vi "TDS - Thermal Desorption Spectroscopy.vi"() -> ()   [LabVIEW 2020]
uses:
  Control 2.ctl
  rga_lv_85/SRSRGA85.llb/SRSRGAo Units Enumeration.ctl
  TDS_ProccesConfig.ctl
  rga_lv_85/SRSRGA85.llb/SRSRGAo RefNum.ctl
  <vilib>/Utility/miscctls.llb/LVRowAndColumnTypeDef.ctl
  <vilib>/Utility/sysdir.llb/System Directory Type.ctl
  <vilib>/Modbus/master/Create Master Instance (TCP).vi
  <vilib>/Utility/config.llb/Read Key (String).vi
  <vilib>/Waveform/WDTFileIO.llb/Export Waveforms To Spreadsheet File (1D).vi
  <vilib>/Utility/config.llb/Write Key (String).vi
  <vilib>/Modbus/master/Modbus Master.lvclass
  <vilib>/Utility/config.llb/NI_LVConfig.lvlib
panel:
  in  "TDS 2":T1={"Target Temp:"=10.0, "Target Ramp:"=1.0, "Ramp unit:"=1, "Temp. unit:"=0, "Target Ue [V]:"=500.0, "Target Ic [A]:"=2.0, "Heating Mode:"=FALSE, "PID Output:"=FALSE, "Regulation Type"=FALSE, "RGA Specifications"=[{"Mass"=2, "Noise Floor"=4, "CEM "=FALSE}], "Heating Recipe"=[]} {"RGA Specifications"."Noise Floor" min=0 max=7; "RGA Specifications"."Mass" min=1 max=300; "Temp. unit:" items=["K"=1, "C"=0]; "Ramp unit:" items=["/s", "/m", "/h"]}
  in  "TDS":T1={"Target Temp:"=10.0, "Target Ramp:"=1.0, "Ramp unit:"=1, "Temp. unit:"=0, "Target Ue [V]:"=500.0, "Target Ic [A]:"=2.0, "Heating Mode:"=FALSE, "PID Output:"=FALSE, "Regulation Type"=FALSE, "RGA Specifications"=[{"Mass"=2, "Noise Floor"=4, "CEM "=FALSE}], "Heating Recipe"=[]} {"RGA Specifications"."Noise Floor" min=0 max=7; "RGA Specifications"."Mass" min=1 max=300; "Temp. unit:" items=["K"=1, "C"=0]; "Ramp unit:" items=["/s", "/m", "/h"]}
  in  "Reconnect":bool
  out "Remote:":bool
  out "RGA_LastData":sgl[](array[numeric]) format="%.2f"
  out "heat_LastData":dbl[](array[numeric])
  out "size(s) 3":i32
  out "HEAT start time":timestamp=timestamp(3621395400.2120705 s since 1904-01-01)
  out "Label.Text":string="D"
  out "Array 2":waveform(dbl)[](array[waveform])
  out "output array":sgl[][](array[numeric])=[[8.752041e-08, 0.0, 0.0, 0.0]]
  out "size(s)":i32=5
  out "Boolean":T2=TRUE
  out "output cluster":T3={"Time"=[0.0, 2.0, 4.0, 6.0, 8.0, 10.0, 12.0, 14.0, 16.0], "Temp"=[24.090000000000032, 10.0, 10.0, 20.0, 20.0, 30.0, 30.0, 40.0, 40.0], "Ramp"=[60.0, 7.045000000000016, 60.0, 5.0, 60.0, 5.0, 60.0, 5.0, 60.0]}
  out "StartTime":timestamp=timestamp(3621394478.675983 s since 1904-01-01)
  out "stopped_loops":bool=TRUE
  in  "Tab Control":T4(tab)
  in  "Start 1":bool=TRUE
  in  "Clear ALL":bool
  out "Waveform Graph":waveform(dbl)[](graph)=[{"t0"=timestamp(3717656497.7127247 s since 1904-01-01), "dt"=0.2, "Y"=array[417 elements]}, {"t0"=timestamp(3717656497.7127247 s since 1904-01-01), "dt"=0.2, "Y"=array[417 elements]}, {"t0"=timestamp(3717656497.7127247 s since 1904-01-01), "dt"=0.2, "Y"=[0.0, 0.0, 0.0, 0.0, 0.0, 0.0, 0.0, 0.0, 0.0, 0.0, 0.0, 0.0, 0.0, 0.0, 0.0, 0.0, 0.0, 0.0, 0.0, 0.0, 0.0, 0.0, 0.0, 0.0, 0.0, 0.0, 0.0, 0.0, 0.0, 0.0, 0.0, 0.0, 0.0, 0.0, 0.0, 0.0, 0.0, 0.0, 0.0, 0.0, 0.0, 0.0, 0.0, 0.0, 0.0, 0.0, 0.0, 0.0, 0.0, 0.0, 0.0, 0.0, 0.0, 0.0, 0.0, 0.0, 0.0, 0.0, 0.0, 0.0, 0.0, 0.0, 0.0, 0.0, 0.0, 0.0, 0.0, 0.0, 0.0, 0.0, 0.0, 0.0, 0.0, 0.0, 0.0, 0.0, 0.0, 0.0, 0.0, 0.0, 0.0, 0.0, 0.0, 0.0, 0.0, 0.0, 0.0, 0.0, 0.0, 0.0, 0.0, 0.0, 0.0, 0.0, 0.0, 0.0, 0.0, 0.0, 0.0, 0.0, 0.0, 0.0, 0.0, 0.0, 0.0, 0.0, 0.0, 0.0, 0.0, 0.0, 0.0, 0.0, 0.0, 0.0, 0.0, 0.0, 0.0, 0.0, 0.0, 0.0, 0.0, 0.0, 0.0, 0.0, 0.0, 0.0, 0.0, 0.0, 0.0, 0.0, 0.0, 0.0, 0.0, 0.0, 0.0, 0.0, 0.0, 0.0, 0.0, 0.0, 0.0, 0.0, 0.0, 0.0, 0.0, 0.0, 0.0, 0.0, 0.0, 0.0, 0.0, 0.0, 0.0, 0.0, 0.0, 0.0, 0.0, 0.0, 0.0, 0.0, 0.0, 0.0, 0.0, 0.0, 0.0, 0.0, 0.0, 0.0, 0.0, 0.0, 0.0, 0.0, 0.0, 0.0, 0.0, 0.0, 0.0, 0.0, 0.0, 0.0, 0.0, 0.0, 0.0, 0.0, 0.0, 0.0, 0.0, 0.0, 0.0, 0.0, 0.0, 0.0, 0.0, 0.0, 0.0, 0.0, 0.0, 0.0, 0.0, 0.0, 0.0, 0.0, 0.0, 0.0, 0.0, 0.0, 0.0, 0.0, 0.0, 0.0, 0.0, 0.0, 0.0, 0.0, 0.0, 0.0, 0.0, 0.0, 0.0, 0.0, 0.0, 0.0, 0.0, 0.0, 0.0, 0.0, 0.0, 0.0, 0.0, 0.0, 0.0, 0.0, 0.0, 0.0, 0.0, 0.0, 0.0, 0.0, 0.0, 0.0, 0.0, 0.0, 0.0, 0.0, 0.0, 0.0, 0.0, 0.0, 0.0, 0.0, 0.0, 0.0, 0.0, 0.0, 0.0, 0.0, 0.0, 0.0, 0.0, 0.0, 0.0, 0.0, 0.0, 0.0, 0.0, 0.0, 0.0, 0.0, 0.0, 0.0, 0.0, 0.0, 0.0, 0.0, 0.0, 0.0, 0.0, 0.0, 0.0, 0.0, 0.0, 0.0, 0.0, 0.0, 0.0, 0.0, 0.0, 0.0, 0.0, 0.0, 0.0, 0.0, 0.0, 0.0, 0.0, 0.0, 0.0, 0.0, 0.0, 0.0, 0.0, 0.0, 0.0, 0.0, 0.0, 0.0, 0.0, 0.0, 0.0, 0.0, 0.0, 0.0, 0.0, 0.0, 0.0, 0.0, 0.0, 0.0, 0.0, 0.0, 0.0, 0.0, 0.0, 0.0, 0.0, 0.0, 0.0, 0.0, 0.0, 0.0, 0.0, 0.0, 0.0, 0.0, 0.0, 0.0, 0.0, 0.0, 0.0, 0.0, 0.0, 0.0, 0.0, 0.0, 0.0, 0.0, 0.0, 0.0, 0.0, 0.0, 0.0, 0.0, 0.0, 0.0, 0.0, 0.0, 0.0, 0.0, 0.0, 0.0, 0.0, 0.0, 0.0, 0.0, 0.0, 0.0, 0.0, 0.0, 0.0, 0.0, 0.0, 0.0, 0.0, 0.0, 0.0, 0.0, 0.0, 0.0, 0.0, 0.0, 0.0, 0.0, 0.0, 0.0, 0.0, 0.0, 0.0, 0.0, 0.0, 0.0, 0.0, 0.0, 0.0, 0.0, 0.0, 0.0, 0.0, 0.0, 0.0, 0.0, 0.0, 0.0, 0.0, 0.0, 0.0, 0.0, 0.0, 0.0, 0.0, 0.0, 0.0, 0.0, 0.0, 0.0, 0.0, 0.0, 0.0]}, {"t0"=timestamp(3717656497.7127247 s since 1904-01-01), "dt"=0.2, "Y"=[0.0, 0.0, 0.0, 0.0, 0.0, 0.0, 0.0, 0.0, 0.0, 0.0, 0.0, 0.0, 0.0, 0.0, 0.0, 0.0, 0.0, 0.0, 0.0, 0.0, 0.0, 0.0, 0.0, 0.0, 0.0, 0.0, 0.0, 0.0, 0.0, 0.0, 0.0, 0.0, 0.0, 0.0, 0.0, 0.0, 0.0, 0.0, 0.0, 0.0, 0.0, 0.0, 0.0, 0.0, 0.0, 0.0, 0.0, 0.0, 0.0, 0.0, 0.0, 0.0, 0.0, 0.0, 0.0, 0.0, 0.0, 0.0, 0.0, 0.0, 0.0, 0.0, 0.0, 0.0, 0.0, 0.0, 0.0, 0.0, 0.0, 0.0, 0.0, 0.0, 0.0, 0.0, 0.0, 0.0, 0.0, 0.0, 0.0, 0.0, 0.0, 0.0, 0.0, 0.0, 0.0, 0.0, 0.0, 0.0, 0.0, 0.0, 0.0, 0.0, 0.0, 0.0, 0.0, 0.0, 0.0, 0.0, 0.0, 0.0, 0.0, 0.0, 0.0, 0.0, 0.0, 0.0, 0.0, 0.0, 0.0, 0.0, 0.0, 0.0, 0.0, 0.0, 0.0, 0.0, 0.0, 0.0, 0.0, 0.0, 0.0, 0.0, 0.0, 0.0, 0.0, 0.0, 0.0, 0.0, 0.0, 0.0, 0.0, 0.0, 0.0, 0.0, 0.0, 0.0, 0.0, 0.0, 0.0, 0.0, 0.0, 0.0, 0.0, 0.0, 0.0, 0.0, 0.0, 0.0, 0.0, 0.0, 0.0, 0.0, 0.0, 0.0, 0.0, 0.0, 0.0, 0.0, 0.0, 0.0, 0.0, 0.0, 0.0, 0.0, 0.0, 0.0, 0.0, 0.0, 0.0, 0.0, 0.0, 0.0, 0.0, 0.0, 0.0, 0.0, 0.0, 0.0, 0.0, 0.0, 0.0, 0.0, 0.0, 0.0, 0.0, 0.0, 0.0, 0.0, 0.0, 0.0, 0.0, 0.0, 0.0, 0.0, 0.0, 0.0, 0.0, 0.0, 0.0, 0.0, 0.0, 0.0, 0.0, 0.0, 0.0, 0.0, 0.0, 0.0, 0.0, 0.0, 0.0, 0.0, 0.0, 0.0, 0.0, 0.0, 0.0, 0.0, 0.0, 0.0, 0.0, 0.0, 0.0, 0.0, 0.0, 0.0, 0.0, 0.0, 0.0, 0.0, 0.0, 0.0, 0.0, 0.0, 0.0, 0.0, 0.0, 0.0, 0.0, 0.0, 0.0, 0.0, 0.0, 0.0, 0.0, 0.0, 0.0, 0.0, 0.0, 0.0, 0.0, 0.0, 0.0, 0.0, 0.0, 0.0, 0.0, 0.0, 0.0, 0.0, 0.0, 0.0, 0.0, 0.0, 0.0, 0.0, 0.0, 0.0, 0.0, 0.0, 0.0, 0.0, 0.0, 0.0, 0.0, 0.0, 0.0, 0.0, 0.0, 0.0, 0.0, 0.0, 0.0, 0.0, 0.0, 0.0, 0.0, 0.0, 0.0, 0.0, 0.0, 0.0, 0.0, 0.0, 0.0, 0.0, 0.0, 0.0, 0.0, 0.0, 0.0, 0.0, 0.0, 0.0, 0.0, 0.0, 0.0, 0.0, 0.0, 0.0, 0.0, 0.0, 0.0, 0.0, 0.0, 0.0, 0.0, 0.0, 0.0, 0.0, 0.0, 0.0, 0.0, 0.0, 0.0, 0.0, 0.0, 0.0, 0.0, 0.0, 0.0, 0.0, 0.0, 0.0, 0.0, 0.0, 0.0, 0.0, 0.0, 0.0, 0.0, 0.0, 0.0, 0.0, 0.0, 0.0, 0.0, 0.0, 0.0, 0.0, 0.0, 0.0, 0.0, 0.0, 0.0, 0.0, 0.0, 0.0, 0.0, 0.0, 0.0, 0.0, 0.0, 0.0, 0.0, 0.0, 0.0, 0.0, 0.0, 0.0, 0.0, 0.0, 0.0, 0.0, 0.0, 0.0, 0.0, 0.0, 0.0, 0.0, 0.0, 0.0, 0.0, 0.0, 0.0, 0.0, 0.0, 0.0, 0.0, 0.0, 0.0, 0.0, 0.0, 0.0, 0.0, 0.0, 0.0, 0.0, 0.0, 0.0, 0.0, 0.0, 0.0, 0.0, 0.0, 0.0, 0.0, 0.0, 0.0, 0.0, 0.0, 0.0, 0.0, 0.0, 0.0, 0.0, 0.0]}, {"t0"=timestamp(3717656497.7127247 s since 1904-01-01), "dt"=0.2, "Y"=[0.0, 0.0, 0.0, 0.0, 0.0, 0.0, 0.0, 0.0, 0.0, 0.0, 0.0, 0.0, 0.0, 0.0, 0.0, 0.0, 0.0, 0.0, 0.0, 0.0, 0.0, 0.0, 0.0, 0.0, 0.0, 0.0, 0.0, 0.0, 0.0, 0.0, 0.0, 0.0, 0.0, 0.0, 0.0, 0.0, 0.0, 0.0, 0.0, 0.0, 0.0, 0.0, 0.0, 0.0, 0.0, 0.0, 0.0, 0.0, 0.0, 0.0, 0.0, 0.0, 0.0, 0.0, 0.0, 0.0, 0.0, 0.0, 0.0, 0.0, 0.0, 0.0, 0.0, 0.0, 0.0, 0.0, 0.0, 0.0, 0.0, 0.0, 0.0, 0.0, 0.0, 0.0, 0.0, 0.0, 0.0, 0.0, 0.0, 0.0, 0.0, 0.0, 0.0, 0.0, 0.0, 0.0, 0.0, 0.0, 0.0, 0.0, 0.0, 0.0, 0.0, 0.0, 0.0, 0.0, 0.0, 0.0, 0.0, 0.0, 0.0, 0.0, 0.0, 0.0, 0.0, 0.0, 0.0, 0.0, 0.0, 0.0, 0.0, 0.0, 0.0, 0.0, 0.0, 0.0, 0.0, 0.0, 0.0, 0.0, 0.0, 0.0, 0.0, 0.0, 0.0, 0.0, 0.0, 0.0, 0.0, 0.0, 0.0, 0.0, 0.0, 0.0, 0.0, 0.0, 0.0, 0.0, 0.0, 0.0, 0.0, 0.0, 0.0, 0.0, 0.0, 0.0, 0.0, 0.0, 0.0, 0.0, 0.0, 0.0, 0.0, 0.0, 0.0, 0.0, 0.0, 0.0, 0.0, 0.0, 0.0, 0.0, 0.0, 0.0, 0.0, 0.0, 0.0, 0.0, 0.0, 0.0, 0.0, 0.0, 0.0, 0.0, 0.0, 0.0, 0.0, 0.0, 0.0, 0.0, 0.0, 0.0, 0.0, 0.0, 0.0, 0.0, 0.0, 0.0, 0.0, 0.0, 0.0, 0.0, 0.0, 0.0, 0.0, 0.0, 0.0, 0.0, 0.0, 0.0, 0.0, 0.0, 0.0, 0.0, 0.0, 0.0, 0.0, 0.0, 0.0, 0.0, 0.0, 0.0, 0.0, 0.0, 0.0, 0.0, 0.0, 0.0, 0.0, 0.0, 0.0, 0.0, 0.0, 0.0, 0.0, 0.0, 0.0, 0.0, 0.0, 0.0, 0.0, 0.0, 0.0, 0.0, 0.0, 0.0, 0.0, 0.0, 0.0, 0.0, 0.0, 0.0, 0.0, 0.0, 0.0, 0.0, 0.0, 0.0, 0.0, 0.0, 0.0, 0.0, 0.0, 0.0, 0.0, 0.0, 0.0, 0.0, 0.0, 0.0, 0.0, 0.0, 0.0, 0.0, 0.0, 0.0, 0.0, 0.0, 0.0, 0.0, 0.0, 0.0, 0.0, 0.0, 0.0, 0.0, 0.0, 0.0, 0.0, 0.0, 0.0, 0.0, 0.0, 0.0, 0.0, 0.0, 0.0, 0.0, 0.0, 0.0, 0.0, 0.0, 0.0, 0.0, 0.0, 0.0, 0.0, 0.0, 0.0, 0.0, 0.0, 0.0, 0.0, 0.0, 0.0, 0.0, 0.0, 0.0, 0.0, 0.0, 0.0, 0.0, 0.0, 0.0, 0.0, 0.0, 0.0, 0.0, 0.0, 0.0, 0.0, 0.0, 0.0, 0.0, 0.0, 0.0, 0.0, 0.0, 0.0, 0.0, 0.0, 0.0, 0.0, 0.0, 0.0, 0.0, 0.0, 0.0, 0.0, 0.0, 0.0, 0.0, 0.0, 0.0, 0.0, 0.0, 0.0, 0.0, 0.0, 0.0, 0.0, 0.0, 0.0, 0.0, 0.0, 0.0, 0.0, 0.0, 0.0, 0.0, 0.0, 0.0, 0.0, 0.0, 0.0, 0.0, 0.0, 0.0, 0.0, 0.0, 0.0, 0.0, 0.0, 0.0, 0.0, 0.0, 0.0, 0.0, 0.0, 0.0, 0.0, 0.0, 0.0, 0.0, 0.0, 0.0, 0.0, 0.0, 0.0, 0.0, 0.0, 0.0, 0.0, 0.0, 0.0, 0.0, 0.0, 0.0, 0.0, 0.0, 0.0, 0.0, 0.0, 0.0, 0.0, 0.0, 0.0, 0.0, 0.0, 0.0, 0.0, 0.0, 0.0, 0.0, 0.0, 0.0, 0.0]}, {"t0"=timestamp(3717656497.7127247 s since 1904-01-01), "dt"=0.2, "Y"=[0.0, 0.0, 0.0, 0.0, 0.0, 0.0, 0.0, 0.0, 0.0, 0.0, 0.0, 0.0, 0.0, 0.0, 0.0, 0.0, 0.0, 0.0, 0.0, 0.0, 0.0, 0.0, 0.0, 0.0, 0.0, 0.0, 0.0, 0.0, 0.0, 0.0, 0.0, 0.0, 0.0, 0.0, 0.0, 0.0, 0.0, 0.0, 0.0, 0.0, 0.0, 0.0, 0.0, 0.0, 0.0, 0.0, 0.0, 0.0, 0.0, 0.0, 0.0, 0.0, 0.0, 0.0, 0.0, 0.0, 0.0, 0.0, 0.0, 0.0, 0.0, 0.0, 0.0, 0.0, 0.0, 0.0, 0.0, 0.0, 0.0, 0.0, 0.0, 0.0, 0.0, 0.0, 0.0, 0.0, 0.0, 0.0, 0.0, 0.0, 0.0, 0.0, 0.0, 0.0, 0.0, 0.0, 0.0, 0.0, 0.0, 0.0, 0.0, 0.0, 0.0, 0.0, 0.0, 0.0, 0.0, 0.0, 0.0, 0.0, 0.0, 0.0, 0.0, 0.0, 0.0, 0.0, 0.0, 0.0, 0.0, 0.0, 0.0, 0.0, 0.0, 0.0, 0.0, 0.0, 0.0, 0.0, 0.0, 0.0, 0.0, 0.0, 0.0, 0.0, 0.0, 0.0, 0.0, 0.0, 0.0, 0.0, 0.0, 0.0, 0.0, 0.0, 0.0, 0.0, 0.0, 0.0, 0.0, 0.0, 0.0, 0.0, 0.0, 0.0, 0.0, 0.0, 0.0, 0.0, 0.0, 0.0, 0.0, 0.0, 0.0, 0.0, 0.0, 0.0, 0.0, 0.0, 0.0, 0.0, 0.0, 0.0, 0.0, 0.0, 0.0, 0.0, 0.0, 0.0, 0.0, 0.0, 0.0, 0.0, 0.0, 0.0, 0.0, 0.0, 0.0, 0.0, 0.0, 0.0, 0.0, 0.0, 0.0, 0.0, 0.0, 0.0, 0.0, 0.0, 0.0, 0.0, 0.0, 0.0, 0.0, 0.0, 0.0, 0.0, 0.0, 0.0, 0.0, 0.0, 0.0, 0.0, 0.0, 0.0, 0.0, 0.0, 0.0, 0.0, 0.0, 0.0, 0.0, 0.0, 0.0, 0.0, 0.0, 0.0, 0.0, 0.0, 0.0, 0.0, 0.0, 0.0, 0.0, 0.0, 0.0, 0.0, 0.0, 0.0, 0.0, 0.0, 0.0, 0.0, 0.0, 0.0, 0.0, 0.0, 0.0, 0.0, 0.0, 0.0, 0.0, 0.0, 0.0, 0.0, 0.0, 0.0, 0.0, 0.0, 0.0, 0.0, 0.0, 0.0, 0.0, 0.0, 0.0, 0.0, 0.0, 0.0, 0.0, 0.0, 0.0, 0.0, 0.0, 0.0, 0.0, 0.0, 0.0, 0.0, 0.0, 0.0, 0.0, 0.0, 0.0, 0.0, 0.0, 0.0, 0.0, 0.0, 0.0, 0.0, 0.0, 0.0, 0.0, 0.0, 0.0, 0.0, 0.0, 0.0, 0.0, 0.0, 0.0, 0.0, 0.0, 0.0, 0.0, 0.0, 0.0, 0.0, 0.0, 0.0, 0.0, 0.0, 0.0, 0.0, 0.0, 0.0, 0.0, 0.0, 0.0, 0.0, 0.0, 0.0, 0.0, 0.0, 0.0, 0.0, 0.0, 0.0, 0.0, 0.0, 0.0, 0.0, 0.0, 0.0, 0.0, 0.0, 0.0, 0.0, 0.0, 0.0, 0.0, 0.0, 0.0, 0.0, 0.0, 0.0, 0.0, 0.0, 0.0, 0.0, 0.0, 0.0, 0.0, 0.0, 0.0, 0.0, 0.0, 0.0, 0.0, 0.0, 0.0, 0.0, 0.0, 0.0, 0.0, 0.0, 0.0, 0.0, 0.0, 0.0, 0.0, 0.0, 0.0, 0.0, 0.0, 0.0, 0.0, 0.0, 0.0, 0.0, 0.0, 0.0, 0.0, 0.0, 0.0, 0.0, 0.0, 0.0, 0.0, 0.0, 0.0, 0.0, 0.0, 0.0, 0.0, 0.0, 0.0, 0.0, 0.0, 0.0, 0.0, 0.0, 0.0, 0.0, 0.0, 0.0, 0.0, 0.0, 0.0, 0.0, 0.0, 0.0, 0.0, 0.0, 0.0, 0.0, 0.0, 0.0, 0.0, 0.0, 0.0, 0.0, 0.0, 0.0, 0.0, 0.0, 0.0]}, {"t0"=timestamp(3717656497.7127247 s since 1904-01-01), "dt"=0.2, "Y"=[0.0, 0.0, 0.0, 0.0, 0.0, 0.0, 0.0, 0.0, 0.0, 0.0, 0.0, 0.0, 0.0, 0.0, 0.0, 0.0, 0.0, 0.0, 0.0, 0.0, 0.0, 0.0, 0.0, 0.0, 0.0, 0.0, 0.0, 0.0, 0.0, 0.0, 0.0, 0.0, 0.0, 0.0, 0.0, 0.0, 0.0, 0.0, 0.0, 0.0, 0.0, 0.0, 0.0, 0.0, 0.0, 0.0, 0.0, 0.0, 0.0, 0.0, 0.0, 0.0, 0.0, 0.0, 0.0, 0.0, 0.0, 0.0, 0.0, 0.0, 0.0, 0.0, 0.0, 0.0, 0.0, 0.0, 0.0, 0.0, 0.0, 0.0, 0.0, 0.0, 0.0, 0.0, 0.0, 0.0, 0.0, 0.0, 0.0, 0.0, 0.0, 0.0, 0.0, 0.0, 0.0, 0.0, 0.0, 0.0, 0.0, 0.0, 0.0, 0.0, 0.0, 0.0, 0.0, 0.0, 0.0, 0.0, 0.0, 0.0, 0.0, 0.0, 0.0, 0.0, 0.0, 0.0, 0.0, 0.0, 0.0, 0.0, 0.0, 0.0, 0.0, 0.0, 0.0, 0.0, 0.0, 0.0, 0.0, 0.0, 0.0, 0.0, 0.0, 0.0, 0.0, 0.0, 0.0, 0.0, 0.0, 0.0, 0.0, 0.0, 0.0, 0.0, 0.0, 0.0, 0.0, 0.0, 0.0, 0.0, 0.0, 0.0, 0.0, 0.0, 0.0, 0.0, 0.0, 0.0, 0.0, 0.0, 0.0, 0.0, 0.0, 0.0, 0.0, 0.0, 0.0, 0.0, 0.0, 0.0, 0.0, 0.0, 0.0, 0.0, 0.0, 0.0, 0.0, 0.0, 0.0, 0.0, 0.0, 0.0, 0.0, 0.0, 0.0, 0.0, 0.0, 0.0, 0.0, 0.0, 0.0, 0.0, 0.0, 0.0, 0.0, 0.0, 0.0, 0.0, 0.0, 0.0, 0.0, 0.0, 0.0, 0.0, 0.0, 0.0, 0.0, 0.0, 0.0, 0.0, 0.0, 0.0, 0.0, 0.0, 0.0, 0.0, 0.0, 0.0, 0.0, 0.0, 0.0, 0.0, 0.0, 0.0, 0.0, 0.0, 0.0, 0.0, 0.0, 0.0, 0.0, 0.0, 0.0, 0.0, 0.0, 0.0, 0.0, 0.0, 0.0, 0.0, 0.0, 0.0, 0.0, 0.0, 0.0, 0.0, 0.0, 0.0, 0.0, 0.0, 0.0, 0.0, 0.0, 0.0, 0.0, 0.0, 0.0, 0.0, 0.0, 0.0, 0.0, 0.0, 0.0, 0.0, 0.0, 0.0, 0.0, 0.0, 0.0, 0.0, 0.0, 0.0, 0.0, 0.0, 0.0, 0.0, 0.0, 0.0, 0.0, 0.0, 0.0, 0.0, 0.0, 0.0, 0.0, 0.0, 0.0, 0.0, 0.0, 0.0, 0.0, 0.0, 0.0, 0.0, 0.0, 0.0, 0.0, 0.0, 0.0, 0.0, 0.0, 0.0, 0.0, 0.0, 0.0, 0.0, 0.0, 0.0, 0.0, 0.0, 0.0, 0.0, 0.0, 0.0, 0.0, 0.0, 0.0, 0.0, 0.0, 0.0, 0.0, 0.0, 0.0, 0.0, 0.0, 0.0, 0.0, 0.0, 0.0, 0.0, 0.0, 0.0, 0.0, 0.0, 0.0, 0.0, 0.0, 0.0, 0.0, 0.0, 0.0, 0.0, 0.0, 0.0, 0.0, 0.0, 0.0, 0.0, 0.0, 0.0, 0.0, 0.0, 0.0, 0.0, 0.0, 0.0, 0.0, 0.0, 0.0, 0.0, 0.0, 0.0, 0.0, 0.0, 0.0, 0.0, 0.0, 0.0, 0.0, 0.0, 0.0, 0.0, 0.0, 0.0, 0.0, 0.0, 0.0, 0.0, 0.0, 0.0, 0.0, 0.0, 0.0, 0.0, 0.0, 0.0, 0.0, 0.0, 0.0, 0.0, 0.0, 0.0, 0.0, 0.0, 0.0, 0.0, 0.0, 0.0, 0.0, 0.0, 0.0, 0.0, 0.0, 0.0, 0.0, 0.0, 0.0, 0.0, 0.0, 0.0, 0.0, 0.0, 0.0, 0.0, 0.0, 0.0, 0.0, 0.0, 0.0, 0.0, 0.0, 0.0, 0.0, 0.0, 0.0, 0.0, 0.0]}, {"t0"=timestamp(3717656497.7127247 s since 1904-01-01), "dt"=0.2, "Y"=[0.0, 0.0, 0.0, 0.0, 0.0, 0.0, 0.0, 0.0, 0.0, 0.0, 0.0, 0.0, 0.0, 0.0, 0.0, 0.0, 0.0, 0.0, 0.0, 0.0, 0.0, 0.0, 0.0, 0.0, 0.0, 0.0, 0.0, 0.0, 0.0, 0.0, 0.0, 0.0, 0.0, 0.0, 0.0, 0.0, 0.0, 0.0, 0.0, 0.0, 0.0, 0.0, 0.0, 0.0, 0.0, 0.0, 0.0, 0.0, 0.0, 0.0, 0.0, 0.0, 0.0, 0.0, 0.0, 0.0, 0.0, 0.0, 0.0, 0.0, 0.0, 0.0, 0.0, 0.0, 0.0, 0.0, 0.0, 0.0, 0.0, 0.0, 0.0, 0.0, 0.0, 0.0, 0.0, 0.0, 0.0, 0.0, 0.0, 0.0, 0.0, 0.0, 0.0, 0.0, 0.0, 0.0, 0.0, 0.0, 0.0, 0.0, 0.0, 0.0, 0.0, 0.0, 0.0, 0.0, 0.0, 0.0, 0.0, 0.0, 0.0, 0.0, 0.0, 0.0, 0.0, 0.0, 0.0, 0.0, 0.0, 0.0, 0.0, 0.0, 0.0, 0.0, 0.0, 0.0, 0.0, 0.0, 0.0, 0.0, 0.0, 0.0, 0.0, 0.0, 0.0, 0.0, 0.0, 0.0, 0.0, 0.0, 0.0, 0.0, 0.0, 0.0, 0.0, 0.0, 0.0, 0.0, 0.0, 0.0, 0.0, 0.0, 0.0, 0.0, 0.0, 0.0, 0.0, 0.0, 0.0, 0.0, 0.0, 0.0, 0.0, 0.0, 0.0, 0.0, 0.0, 0.0, 0.0, 0.0, 0.0, 0.0, 0.0, 0.0, 0.0, 0.0, 0.0, 0.0, 0.0, 0.0, 0.0, 0.0, 0.0, 0.0, 0.0, 0.0, 0.0, 0.0, 0.0, 0.0, 0.0, 0.0, 0.0, 0.0, 0.0, 0.0, 0.0, 0.0, 0.0, 0.0, 0.0, 0.0, 0.0, 0.0, 0.0, 0.0, 0.0, 0.0, 0.0, 0.0, 0.0, 0.0, 0.0, 0.0, 0.0, 0.0, 0.0, 0.0, 0.0, 0.0, 0.0, 0.0, 0.0, 0.0, 0.0, 0.0, 0.0, 0.0, 0.0, 0.0, 0.0, 0.0, 0.0, 0.0, 0.0, 0.0, 0.0, 0.0, 0.0, 0.0, 0.0, 0.0, 0.0, 0.0, 0.0, 0.0, 0.0, 0.0, 0.0, 0.0, 0.0, 0.0, 0.0, 0.0, 0.0, 0.0, 0.0, 0.0, 0.0, 0.0, 0.0, 0.0, 0.0, 0.0, 0.0, 0.0, 0.0, 0.0, 0.0, 0.0, 0.0, 0.0, 0.0, 0.0, 0.0, 0.0, 0.0, 0.0, 0.0, 0.0, 0.0, 0.0, 0.0, 0.0, 0.0, 0.0, 0.0, 0.0, 0.0, 0.0, 0.0, 0.0, 0.0, 0.0, 0.0, 0.0, 0.0, 0.0, 0.0, 0.0, 0.0, 0.0, 0.0, 0.0, 0.0, 0.0, 0.0, 0.0, 0.0, 0.0, 0.0, 0.0, 0.0, 0.0, 0.0, 0.0, 0.0, 0.0, 0.0, 0.0, 0.0, 0.0, 0.0, 0.0, 0.0, 0.0, 0.0, 0.0, 0.0, 0.0, 0.0, 0.0, 0.0, 0.0, 0.0, 0.0, 0.0, 0.0, 0.0, 0.0, 0.0, 0.0, 0.0, 0.0, 0.0, 0.0, 0.0, 0.0, 0.0, 0.0, 0.0, 0.0, 0.0, 0.0, 0.0, 0.0, 0.0, 0.0, 0.0, 0.0, 0.0, 0.0, 0.0, 0.0, 0.0, 0.0, 0.0, 0.0, 0.0, 0.0, 0.0, 0.0, 0.0, 0.0, 0.0, 0.0, 0.0, 0.0, 0.0, 0.0, 0.0, 0.0, 0.0, 0.0, 0.0, 0.0, 0.0, 0.0, 0.0, 0.0, 0.0, 0.0, 0.0, 0.0, 0.0, 0.0, 0.0, 0.0, 0.0, 0.0, 0.0, 0.0, 0.0, 0.0, 0.0, 0.0, 0.0, 0.0, 0.0, 0.0, 0.0, 0.0, 0.0, 0.0, 0.0, 0.0, 0.0, 0.0, 0.0, 0.0, 0.0, 0.0, 0.0, 0.0, 0.0, 0.0, 0.0]}, {"t0"=timestamp(3717656497.7127247 s since 1904-01-01), "dt"=0.2, "Y"=[0.0, 0.0, 0.0, 0.0, 0.0, 0.0, 0.0, 0.0, 0.0, 0.0, 0.0, 0.0, 0.0, 0.0, 0.0, 0.0, 0.0, 0.0, 0.0, 0.0, 0.0, 0.0, 0.0, 0.0, 0.0, 0.0, 0.0, 0.0, 0.0, 0.0, 0.0, 0.0, 0.0, 0.0, 0.0, 0.0, 0.0, 0.0, 0.0, 0.0, 0.0, 0.0, 0.0, 0.0, 0.0, 0.0, 0.0, 0.0, 0.0, 0.0, 0.0, 0.0, 0.0, 0.0, 0.0, 0.0, 0.0, 0.0, 0.0, 0.0, 0.0, 0.0, 0.0, 0.0, 0.0, 0.0, 0.0, 0.0, 0.0, 0.0, 0.0, 0.0, 0.0, 0.0, 0.0, 0.0, 0.0, 0.0, 0.0, 0.0, 0.0, 0.0, 0.0, 0.0, 0.0, 0.0, 0.0, 0.0, 0.0, 0.0, 0.0, 0.0, 0.0, 0.0, 0.0, 0.0, 0.0, 0.0, 0.0, 0.0, 0.0, 0.0, 0.0, 0.0, 0.0, 0.0, 0.0, 0.0, 0.0, 0.0, 0.0, 0.0, 0.0, 0.0, 0.0, 0.0, 0.0, 0.0, 0.0, 0.0, 0.0, 0.0, 0.0, 0.0, 0.0, 0.0, 0.0, 0.0, 0.0, 0.0, 0.0, 0.0, 0.0, 0.0, 0.0, 0.0, 0.0, 0.0, 0.0, 0.0, 0.0, 0.0, 0.0, 0.0, 0.0, 0.0, 0.0, 0.0, 0.0, 0.0, 0.0, 0.0, 0.0, 0.0, 0.0, 0.0, 0.0, 0.0, 0.0, 0.0, 0.0, 0.0, 0.0, 0.0, 0.0, 0.0, 0.0, 0.0, 0.0, 0.0, 0.0, 0.0, 0.0, 0.0, 0.0, 0.0, 0.0, 0.0, 0.0, 0.0, 0.0, 0.0, 0.0, 0.0, 0.0, 0.0, 0.0, 0.0, 0.0, 0.0, 0.0, 0.0, 0.0, 0.0, 0.0, 0.0, 0.0, 0.0, 0.0, 0.0, 0.0, 0.0, 0.0, 0.0, 0.0, 0.0, 0.0, 0.0, 0.0, 0.0, 0.0, 0.0, 0.0, 0.0, 0.0, 0.0, 0.0, 0.0, 0.0, 0.0, 0.0, 0.0, 0.0, 0.0, 0.0, 0.0, 0.0, 0.0, 0.0, 0.0, 0.0, 0.0, 0.0, 0.0, 0.0, 0.0, 0.0, 0.0, 0.0, 0.0, 0.0, 0.0, 0.0, 0.0, 0.0, 0.0, 0.0, 0.0, 0.0, 0.0, 0.0, 0.0, 0.0, 0.0, 0.0, 0.0, 0.0, 0.0, 0.0, 0.0, 0.0, 0.0, 0.0, 0.0, 0.0, 0.0, 0.0, 0.0, 0.0, 0.0, 0.0, 0.0, 0.0, 0.0, 0.0, 0.0, 0.0, 0.0, 0.0, 0.0, 0.0, 0.0, 0.0, 0.0, 0.0, 0.0, 0.0, 0.0, 0.0, 0.0, 0.0, 0.0, 0.0, 0.0, 0.0, 0.0, 0.0, 0.0, 0.0, 0.0, 0.0, 0.0, 0.0, 0.0, 0.0, 0.0, 0.0, 0.0, 0.0, 0.0, 0.0, 0.0, 0.0, 0.0, 0.0, 0.0, 0.0, 0.0, 0.0, 0.0, 0.0, 0.0, 0.0, 0.0, 0.0, 0.0, 0.0, 0.0, 0.0, 0.0, 0.0, 0.0, 0.0, 0.0, 0.0, 0.0, 0.0, 0.0, 0.0, 0.0, 0.0, 0.0, 0.0, 0.0, 0.0, 0.0, 0.0, 0.0, 0.0, 0.0, 0.0, 0.0, 0.0, 0.0, 0.0, 0.0, 0.0, 0.0, 0.0, 0.0, 0.0, 0.0, 0.0, 0.0, 0.0, 0.0, 0.0, 0.0, 0.0, 0.0, 0.0, 0.0, 0.0, 0.0, 0.0, 0.0, 0.0, 0.0, 0.0, 0.0, 0.0, 0.0, 0.0, 0.0, 0.0, 0.0, 0.0, 0.0, 0.0, 0.0, 0.0, 0.0, 0.0, 0.0, 0.0, 0.0, 0.0, 0.0, 0.0, 0.0, 0.0, 0.0, 0.0, 0.0, 0.0, 0.0, 0.0, 0.0, 0.0, 0.0, 0.0, 0.0, 0.0, 0.0, 0.0, 0.0, 0.0]}]
  out "main Graph":T5(graph)={"heat_LastData[0]"=21.230000000000018, "heat_LastData[1]"=-273.15, "heat_LastData[2]"=0.0, "heat_LastData[3]"=0.0, "heat_LastData[4]"=0.0, "heat_LastData[5]"=0.0, "heat_LastData[6]"=0.0, "heat_LastData[7]"=0.0, "heat_LastData[8]"=0.0}
  in  "Start 3":bool=TRUE
  out "XY Graph 2":cluster{dbl[], dbl[]}[](graph)
  in  "Play Button":bool
  in  "Media Stop Button":bool
  in  "Add Step":bool
  in  "Remove STEP":bool
  in  "Remove":bool
  out "XY Graph":cluster{"X":dbl, "Y":dbl}[](graph)=[{"X"=0.0, "Y"=24.090000000000032}, {"X"=2.0, "Y"=10.0}, {"X"=4.0, "Y"=10.0}, {"X"=6.0, "Y"=20.0}, {"X"=8.0, "Y"=20.0}, {"X"=10.0, "Y"=30.0}, {"X"=12.0, "Y"=30.0}, {"X"=14.0, "Y"=40.0}, {"X"=16.0, "Y"=40.0}]
  out "Actual step:":i32
  in  "Pause Button":bool
  in  "Skip Forward Button":bool
  in  "Skip Back Button":bool
  in  "START RGA":bool
  out "Loop Time [ms]":u32=251
  in  "stop 3":bool
  in  "Rate (sec)":dbl=0.25 min=0.001
  out "P vs. t":sgl[][](graph)=[[8.752041e-08, 0.0, 0.0, 0.0]]
  in  "Clear ALL 2":bool
  in  "Start 2":bool=TRUE
  out "main Graph 2":T6(graph)
  in  "Tab Control 2":T7(tab)
  out "Uc Act.: 2":dbl caption="Uc Act.:" format="%#_g V"
  out "Ic Act.: 2":dbl caption="Ic Act.:" format="%#_g A"
  out "Ue Act.: 2":dbl caption="Ue Act.:" format="%#_g V"
  out "Ie Act.: 2":dbl caption="Ie Act.:" format="%#_g mA"
  out "Text Ring 6":u16(ring) items=["K"=1, "C"=0]
  out "Text Ring 5":u16(ring) items=["C/s", "C/m", "C/h"]
  out "Act. Ramp:":dbl=1.0
  out "To next step [s]:":dbl format="%.1f"
  in  "Save As Button":bool
  in  "Regulation TYpe":bool caption="Regulation Type:"
  in  "Target Ue [V]:":dbl=500.0
  in  "Target Ic [A]:":dbl=2.0
  in  "PID Output:":bool caption="PID Output Signal:"
  in  "Heating Mode:":bool
  out "Text Ring 3":u16(ring) items=["C/s", "C/m", "C/h"]
  out "Interlock:":bool
  out "Operate:":bool
  out "Text Ring":u16(ring) items=["K"=1, "C"=0]
  in  "OperateButton":bool caption="Operate:"
  out "Act. Temp:":dbl=24.100000000000023
  out "Act. P":dbl=100.0
  out "Act. I":dbl=50.0
  out "Act. D":dbl=1.0
  in  "Target Temp:":dbl=10.0
  in  "Target Ramp:":dbl=1.0
  out "Act. Setpoint:":dbl=21.55000000000001
  out "Actual step:":i32
  out "Text Ring 2":u16(ring) items=["K"=1, "C"=0]
  out "RES active:":bool
  out "EB active:":bool
  in  "Ramp unit:":u16(ring)=1 items=["/s", "/m", "/h"]
  in  "Temp. unit:":u16(ring) items=["K"=1, "C"=0]
  in  "Channel:":u16(ring)=7 items=["D1"=9, "D2"=11, "RTD"=13, "TC1"=5, "TC2"=7]
  in  "clean":bool
  out "Operate status::":bool[](array[boolean])=[FALSE, FALSE, FALSE, FALSE, FALSE, TRUE, TRUE, TRUE, FALSE, FALSE, FALSE, TRUE, FALSE, FALSE, FALSE, FALSE]
  out "Uc Act.:":dbl
  out "Ic Act.:":dbl
  out "Uc Act.:":dbl
  out "Ic Act.:":dbl
  out "Ue Act.:":dbl
  out "Ie Act.:":dbl
  in  "Ie limit [mA]:":dbl
  in  "Ue limit [V]:":dbl
  in  "Ic limit [A]:":dbl
  in  "Uc limit [V]:":dbl
  in  "Ic limit:1":dbl caption="Ic limit [A]:"
  in  "Uc limit:1":dbl caption="Uc limit [V]:"
  out "New D:":dbl=1.0
  out "New I:":dbl=50.0
  out "New P:":dbl=100.0
  in  "PID auto tab":string[][](table)
  in  "PID manual setting":string[][](table)=[["100", "50", "1"]]
  in  "Auto PID control:":bool=TRUE
  out "New PID request":bool
  in  "Loadproject":bool
  in  "Saveproject":bool
  in  "Sampling time:":dbl=250.0 format="%#_g ms"
  in  "Adv.RampControl":bool=TRUE
  out "Connected:":bool=TRUE
  in  "Reconect":bool
  out "Comunication error:":bool
  out "Text Ring 4":u16(ring) items=["C/s", "C/m", "C/h"]
  out "Loop time:":u32=499
  in  "Lock Button":bool
  in  "Address:":string="192.168.201.50"
  out "error out":T8
  in  "Default Ramp:":dbl=60.0
  out "ResetActRamp":bool
  out "size(s) 2":i32=7
  out "x+y":timestamp[](array[timestamp])=[timestamp(3621394478.675983 s since 1904-01-01), timestamp(3621394598.675983 s since 1904-01-01), timestamp(3621394718.675983 s since 1904-01-01), timestamp(3621394838.675983 s since 1904-01-01), timestamp(3621394958.675983 s since 1904-01-01), timestamp(3621395078.675983 s since 1904-01-01), timestamp(3621395198.675983 s since 1904-01-01), timestamp(3621395318.675983 s since 1904-01-01), timestamp(3621395438.675983 s since 1904-01-01)]
  out "Temperature_Pos_Tab":cluster{"X":dbl, "Y":dbl}[](array[cluster])=[{"X"=0.0, "Y"=24.090000000000032}, {"X"=2.0, "Y"=10.0}, {"X"=4.0, "Y"=10.0}, {"X"=6.0, "Y"=20.0}, {"X"=8.0, "Y"=20.0}, {"X"=10.0, "Y"=30.0}, {"X"=12.0, "Y"=30.0}, {"X"=14.0, "Y"=40.0}, {"X"=16.0, "Y"=40.0}]
  in  "Tab Control 3":enum32{"RGA control", "RGA setting"}(tab)
  out "CEM:":bool
  out "Filament:":bool
  in  "Disconnect":bool
  in  "Connect":bool
  in  "Connection Type:":u16(ring)=1 items=["Ethernet", "Serial"]
  in  "Specifications":T9(array[cluster])=[{"Mass"=2, "Noise Floor"=4, "CEM "=FALSE}] {"Noise Floor" min=0 max=7; "Mass" min=1 max=300}
  in  "Units:":T10
  in  "CEM:":bool
  in  "Filament:":bool
  out "Connected:":bool
  out "Error:":bool
  in  "START RGA  2":bool
  in  "stop 4":bool
  out "Numeric":i32
  in  "Electron Emission [mA]":sgl=1.0 format="%.2f"
  out "Act. Electron Emission":sgl format="%.2f"
  out "Error out:":T11
  in  "ionizer":bool
  in  "detector":bool
  in  "stop":bool=TRUE
  # "RES:"
  # "EB:"
  # "EB:"
  # "Process config.:"
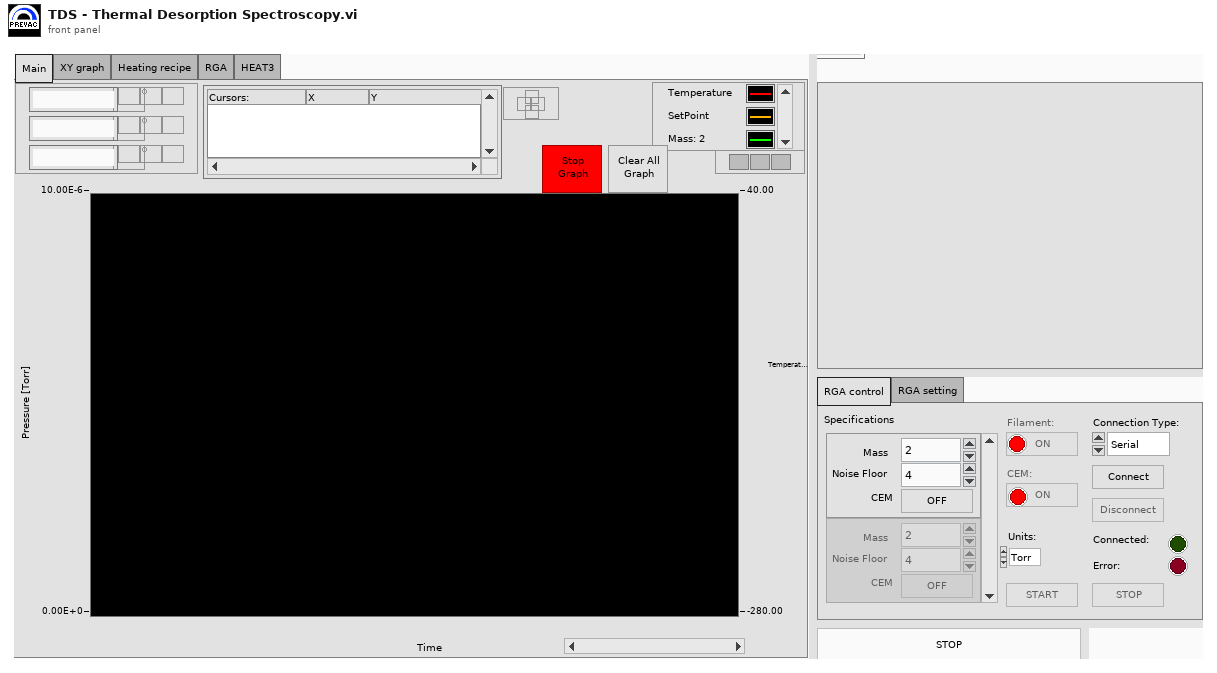
[diagram p1: front panel]
types:
  T1 = typedef "TDS_ProccesConfig.ctl" = cluster{"Target Temp:":dbl, "Target Ramp:":dbl, "Ramp unit:":u16, "Temp. unit:":u16, "Target Ue [V]:":dbl, "Target Ic [A]:":dbl, "Heating Mode:":bool, "PID Output:":bool, "Regulation Type":bool, "RGA Specifications":cluster{"Mass":i32, "Noise Floor":i32, "CEM ":bool}[], "Heating Recipe":cluster{"X":dbl, "Y":dbl}[]}
  T2 = typedef "Control 2.ctl" = bool
  T3 = cluster{"Time":dbl[], "Temp":dbl[], "Ramp":dbl[]}
  T4 = enum32{"Main", "XY graph", "Heating recipe", "RGA", "HEAT3"}
  T5 = cluster{"heat_LastData[0]":dbl, "heat_LastData[1]":dbl, "heat_LastData[2]":dbl, "heat_LastData[3]":dbl, "heat_LastData[4]":dbl, "heat_LastData[5]":dbl, "heat_LastData[6]":dbl, "heat_LastData[7]":dbl, "heat_LastData[8]":dbl}
  T6 = cluster{"[0]":dbl, "[1]":dbl, "[2]":dbl, "[3]":dbl}
  T7 = enum32{"HEAT3 control", "HEAT3 limits", "PID", "HEAT3 configurations"}
  T8 = cluster{"Status:":bool, "Code:":i32, "source":string}
  T9 = cluster{"Mass":i32, "Noise Floor":i32, "CEM ":bool}[]
  T10 = typedef "SRSRGAo Units Enumeration.ctl" = enum16{"Torr", "mTorr", "mbar", "bar", "Pa", "A", "ppm"}
  T11 = cluster{"Status:":bool, "Code:":i32, "Source:":string}
  T12 = typedef "SRSRGAo RefNum.ctl" = u16
  T13 = typedef "LVRowAndColumnTypeDef.ctl" = cluster{"Row":i32, "Column":i32}
  T14 = enum8{"Enabled", "Disabled", "Disabled and Grayed Out"}
  T15 = cluster{"Name":string, "Color":u32, "Style":u8, "Point Style":u8, "Name Visible":bool, "Allow Drag":bool, "Cursor Mode":u32, "Plot":i32, "Index":i32, "Position":cluster{"X":dbl, "Y":dbl}, "X Scale":u32, "Y Scale":u32, "Watch Plots":i32[], "Watch All Plots":bool, "Plot Area":i32, "Label Offset":cluster{"X":dbl, "Y":dbl}}
  T16 = cluster{"heat_LastData[0]":dbl, "heat_LastData[1]":dbl, "heat_LastData[2]":dbl, "heat_LastData[3]":dbl, "heat_LastData[4]":dbl, "heat_LastData[5]":dbl, "heat_LastData[6]":dbl, "heat_LastData[7]":dbl, "heat_LastData[8]":dbl}[]
  T17 = enum16{"open", "replace", "create", "open or create", "replace or create", "replace or create with confirmation"}
  T18 = cluster{"[0]":dbl, "[1]":dbl, "[2]":dbl, "[3]":dbl}[]
  T19 = enum16{"Initialize", "Init+Factory", "Init+Fact+Standby"}
  T20 = typedef "LVRectTypeDef.ctl" = cluster{"Left":i16, "Top":i16, "Right":i16, "Bottom":i16}
  T21 = typedef "NI_LVConfig.lvlib/Config Data RefNum.ctl" = refnum<k1>
  T22 = typedef "LVCursorListTypeDef.ctl" = cluster{"Name":string, "Color":u32, "Style":u8, "Point Style":u8, "Name Visible":bool, "Allow Drag":bool, "Cursor Mode":u32, "Plot":i32, "Index":i32, "Position":cluster{"X":dbl, "Y":dbl}, "X Scale":u32, "Y Scale":u32, "Watch Plots":i32[], "Watch All Plots":bool, "Plot Area":i32, "Label Offset":cluster{"X":dbl, "Y":dbl}}[]
  T23 = typedef "LVPoint32TypeDef.ctl" = cluster{"Horizontal":i32, "Vertical":i32}
  T24 = typedef "LVBoundsTypeDef.ctl" = cluster{"Width":u32, "Height":u32}
  T25 = typedef "LVPositionTypeDef.ctl" = cluster{"Left":i32, "Top":i32}
  T26 = typedef "LVRangeTypeDef.ctl" = cluster{"Minimum":dbl, "Maximum":dbl, "Increment":dbl, "Minor Increment":dbl, "Start":dbl}
  T27 = cluster{"Name":string, "Color":u32, "Style":u8, "Point Style":u8, "Name Visible":bool, "Allow Drag":bool, "Lock Style":u32, "Plot":u32, "Index":i32, "Position":cluster{"X":dbl, "Y":dbl}}[]
  T28 = cluster{"Name":string, "Color":u32, "Style":u8, "Point Style":u8, "Name Visible":bool, "Allow Drag":bool, "Lock Style":u32, "Plot":u32, "Index":i32, "Position":cluster{"X":dbl, "Y":dbl}}
  T29 = cluster{"Name":string, "Color":u32, "Style":u8, "Point Style":u8, "Name Visible":bool, "Allow Drag":bool, "Cursor Mode":u32, "Plot":i32, "Index":i32, "Position":cluster{"X":dbl, "Y":dbl}, "X Scale":u32, "Y Scale":u32, "Watch Plots":i32[], "Watch All Plots":bool, "Plot Area":i32, "Label Offset":cluster{"X":dbl, "Y":dbl}}[]
  T30 = typedef "System Directory Type.ctl" = i32
  T31 = cluster{"Mass":i32, "Noise Floor":i32, "CEM On?":bool}[]
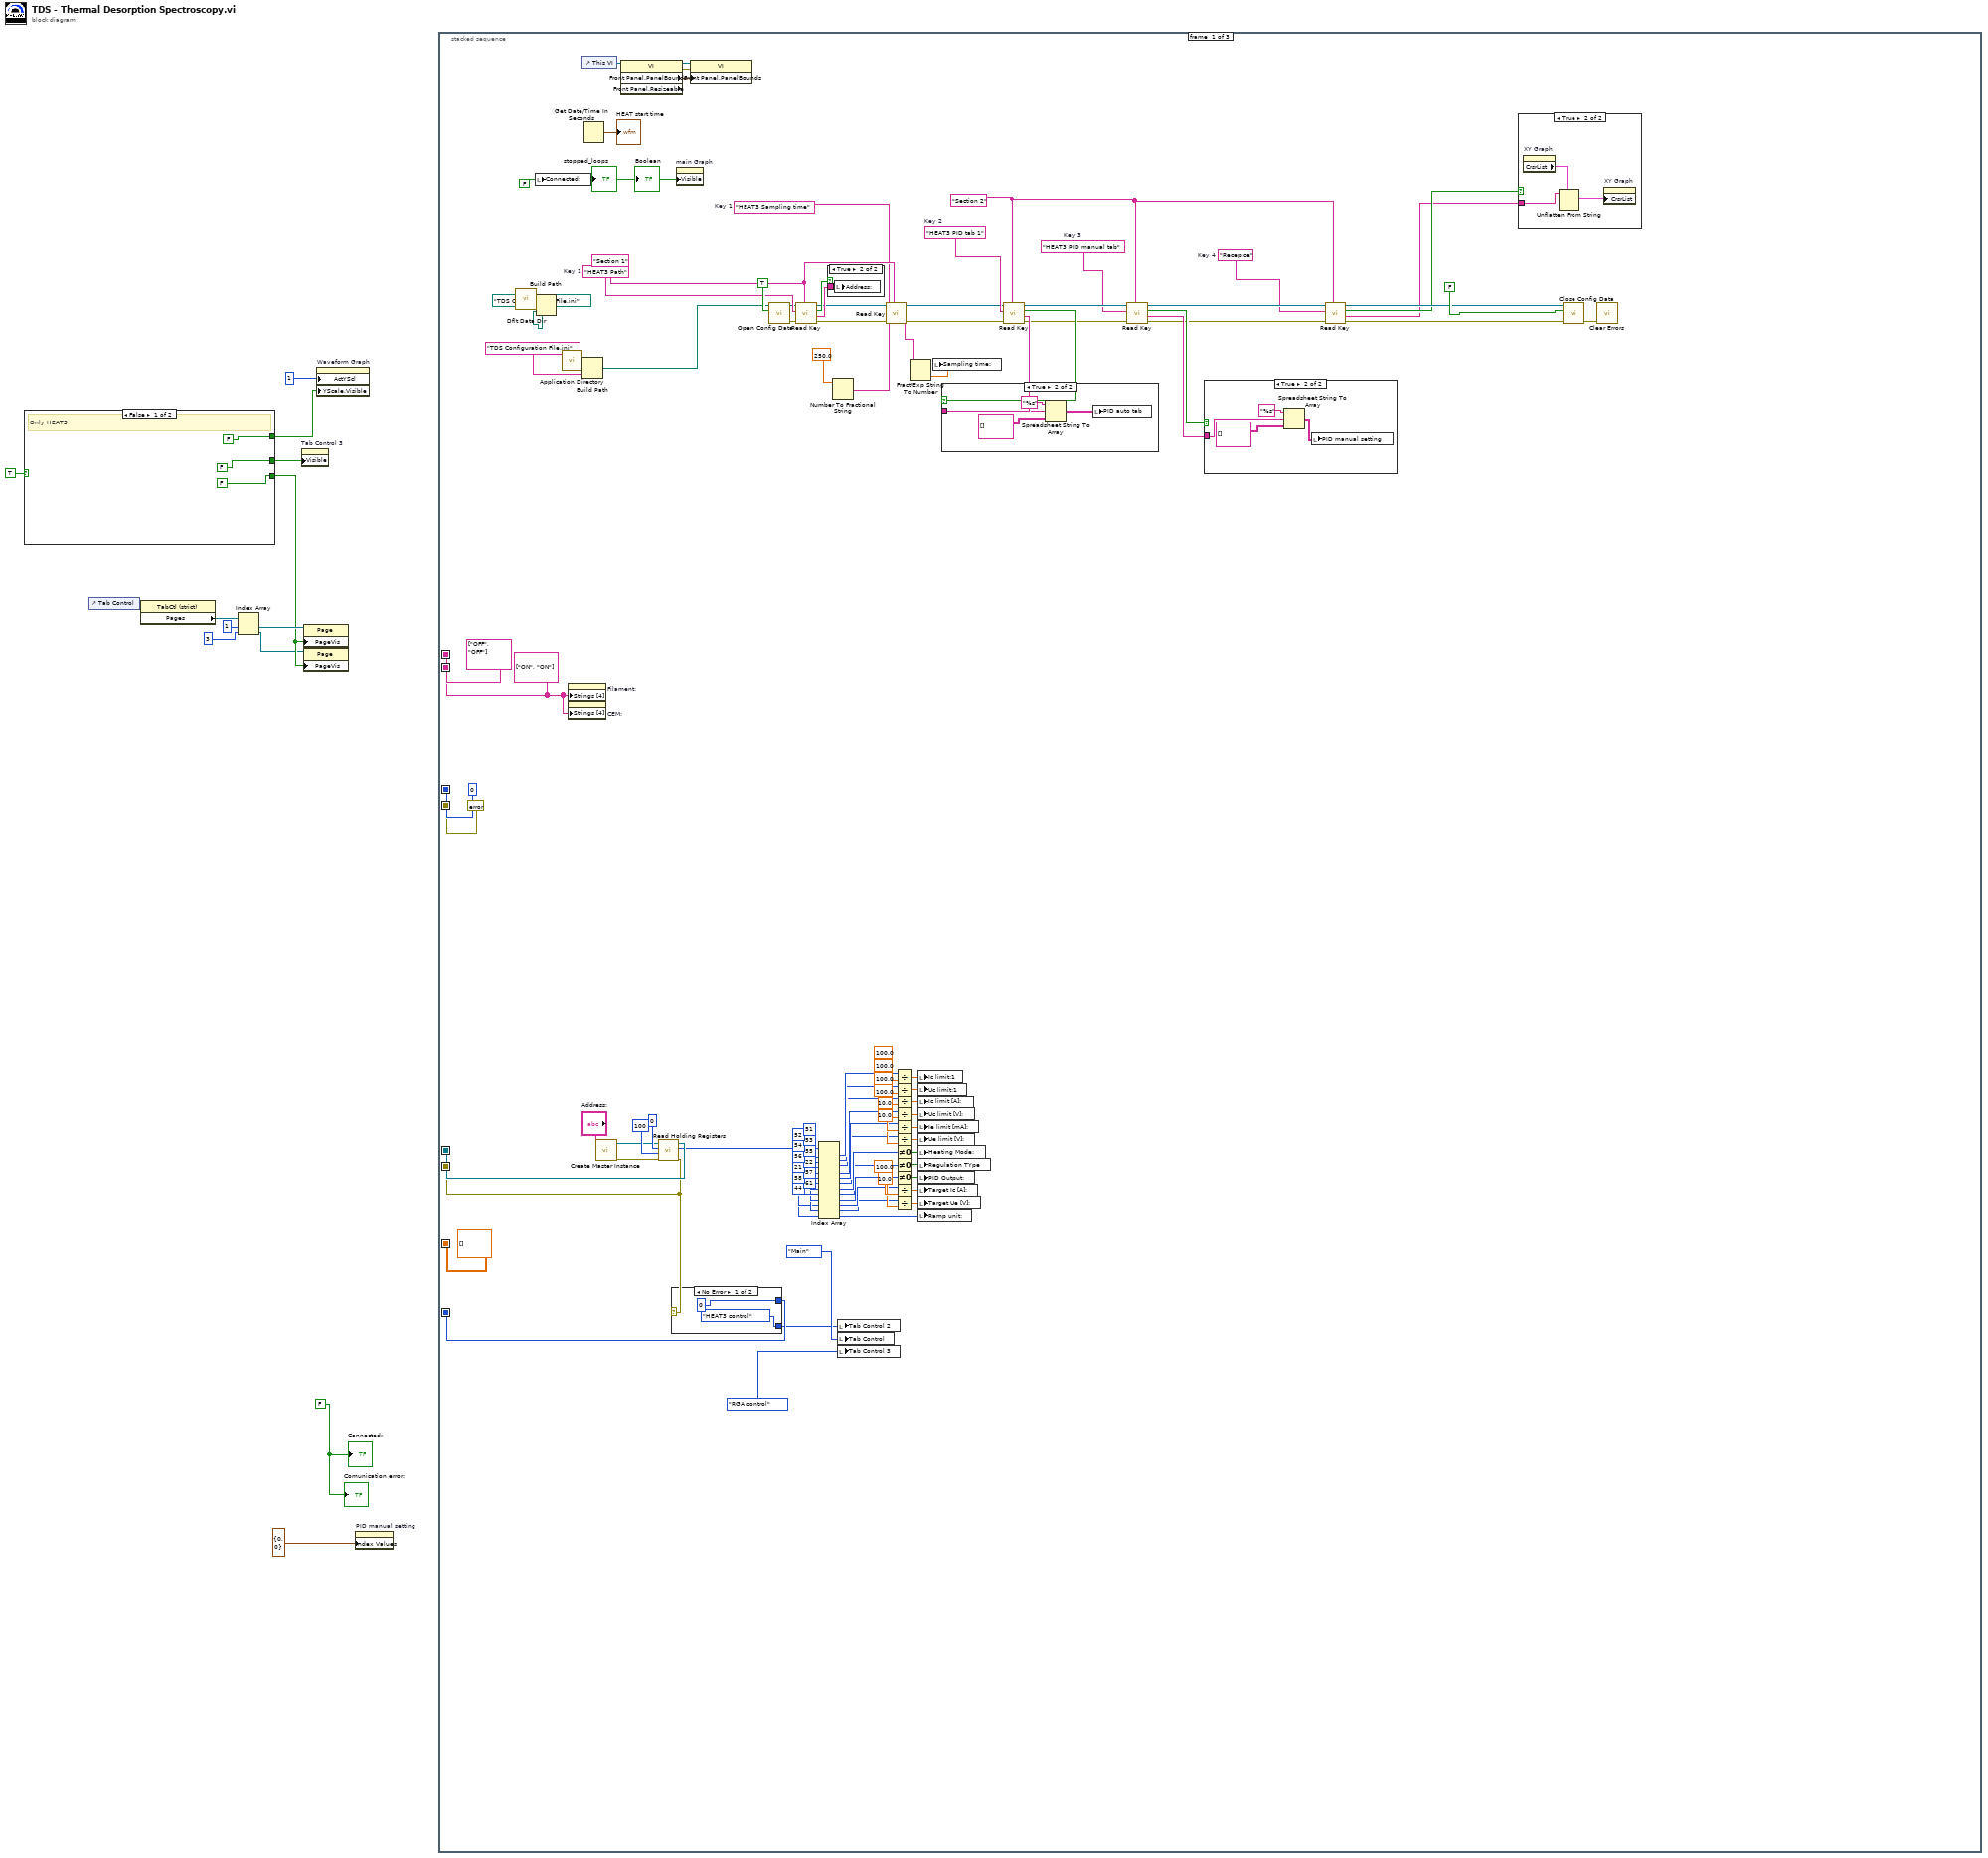
[diagram p0: block diagram]
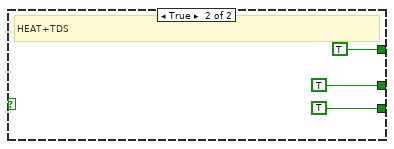
[diagram p2: hidden frame]
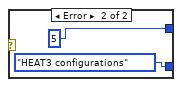
[diagram p6: hidden frame]
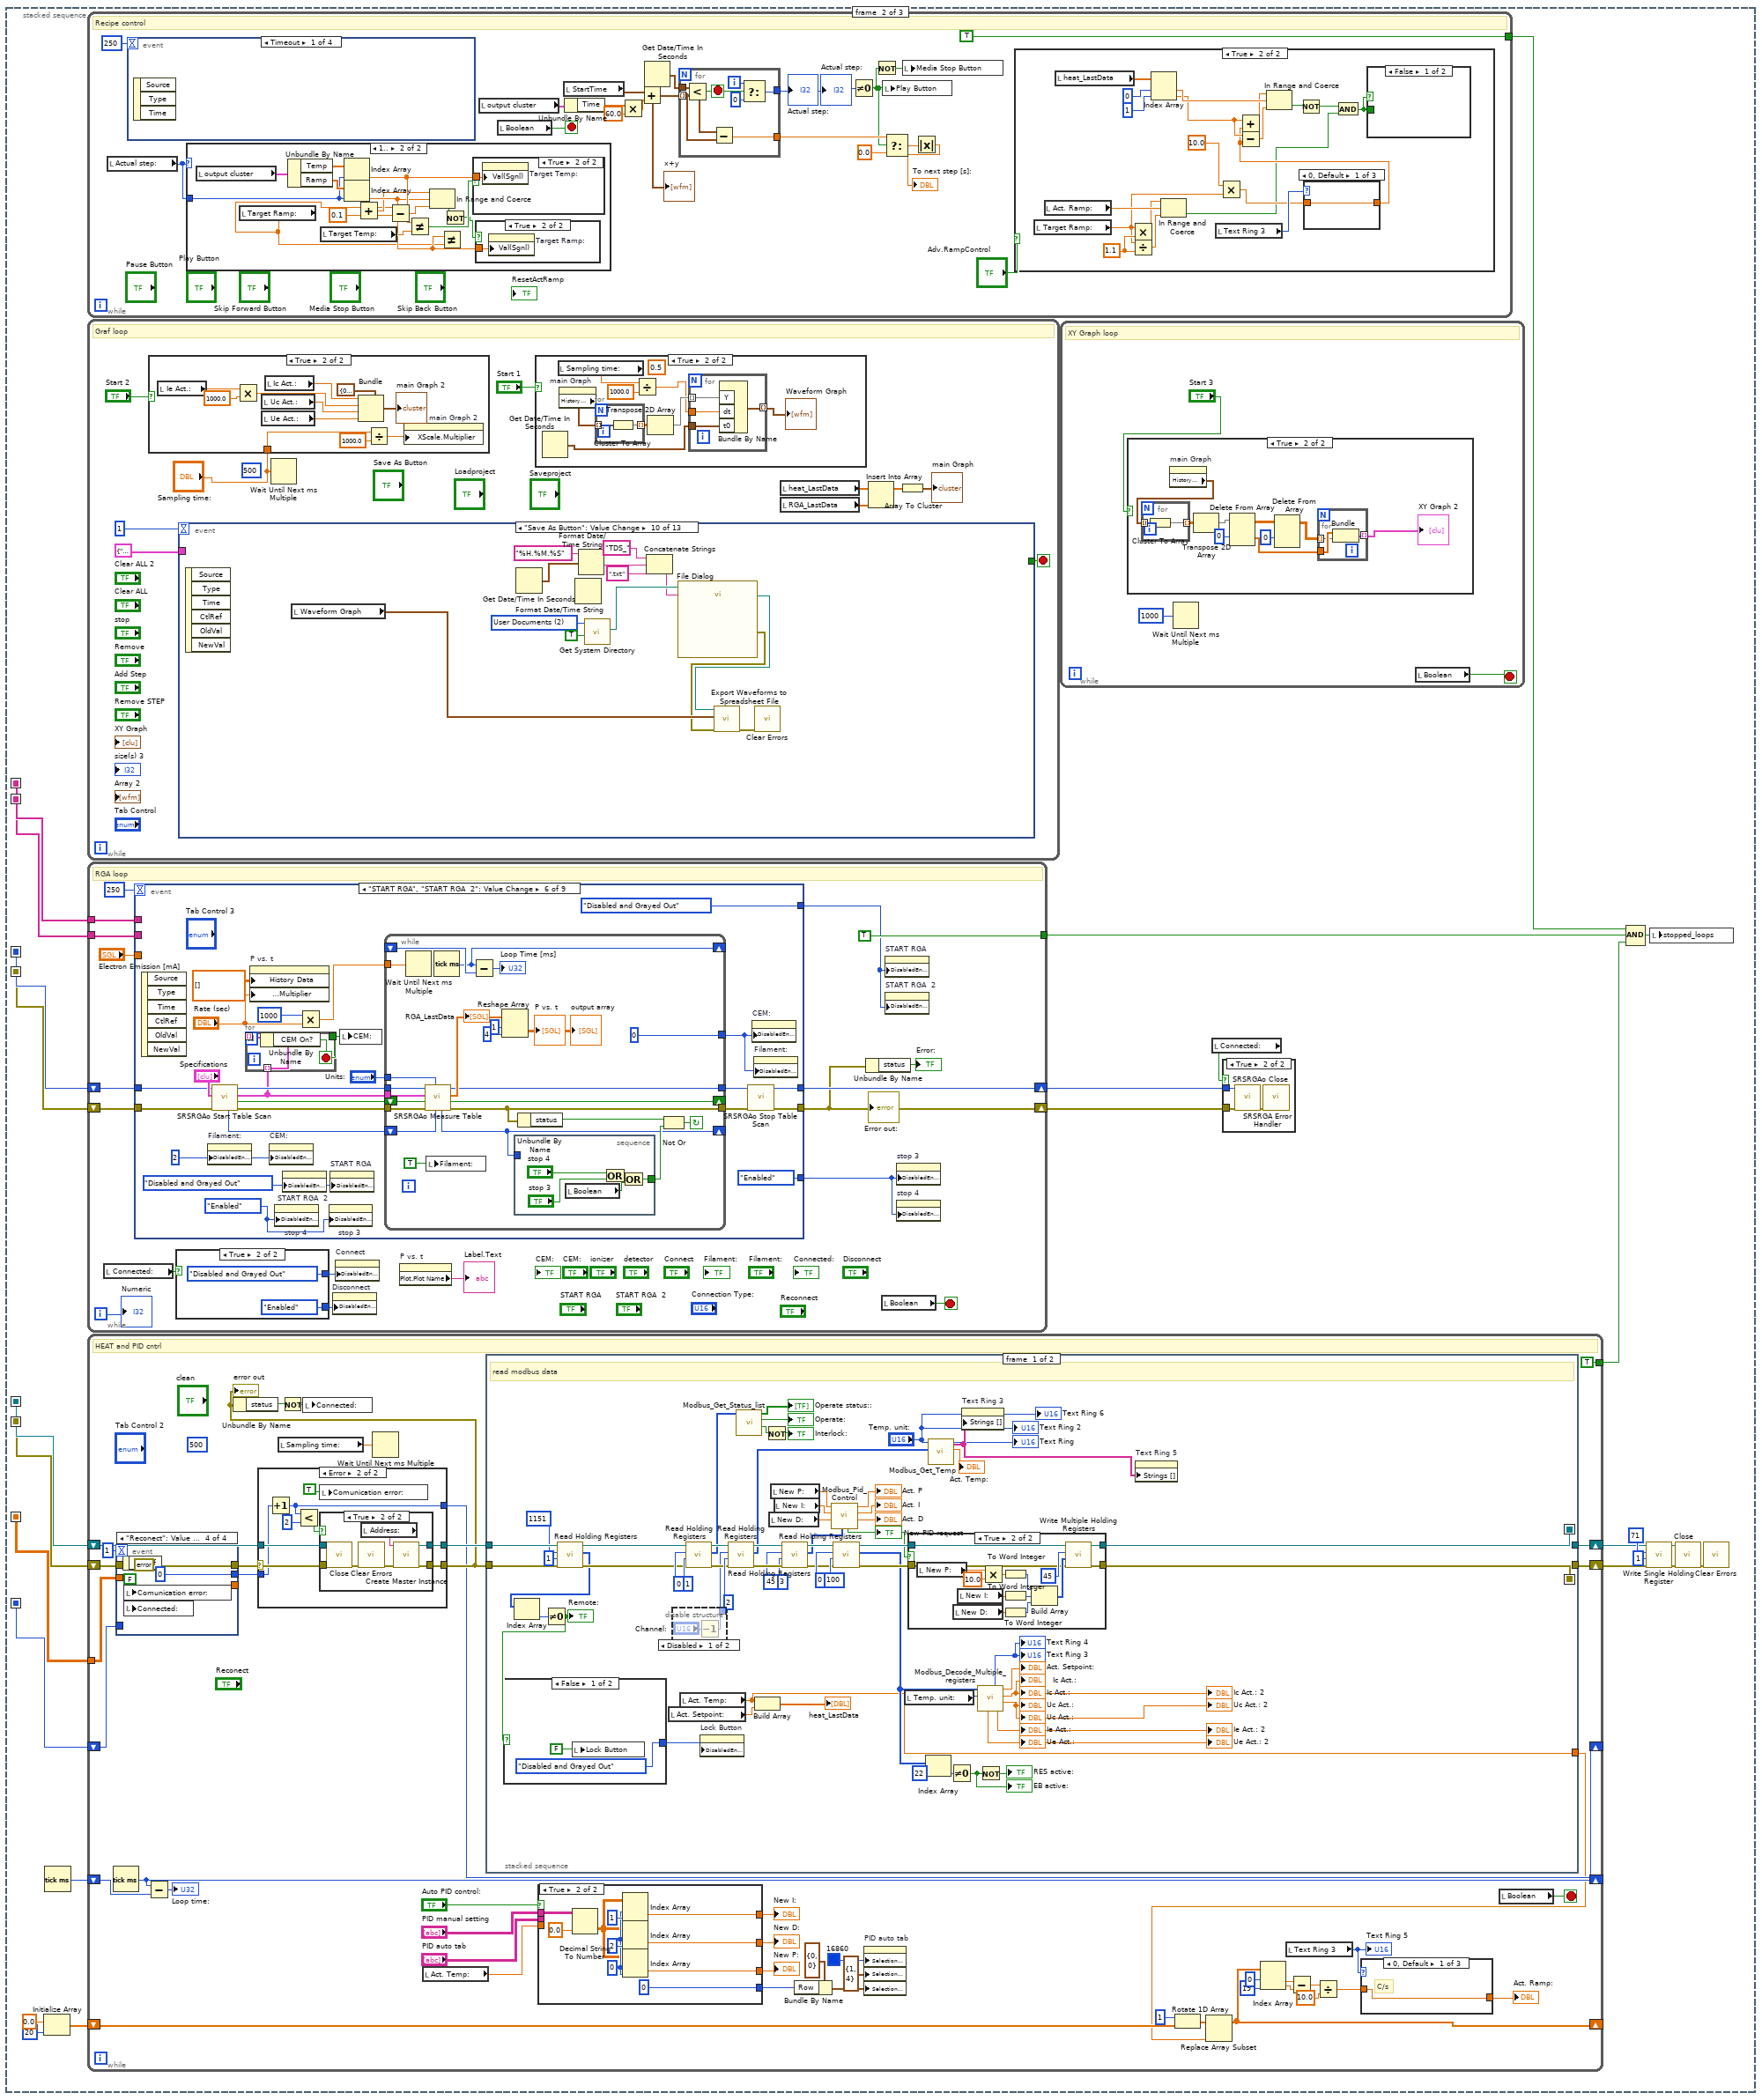
[diagram p8: hidden frame]
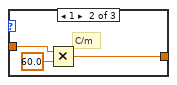
[diagram p11: hidden frame]
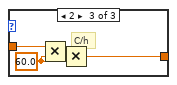
[diagram p12: hidden frame]
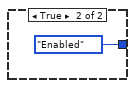
[diagram p13: hidden frame]
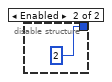
[diagram p14: hidden frame]
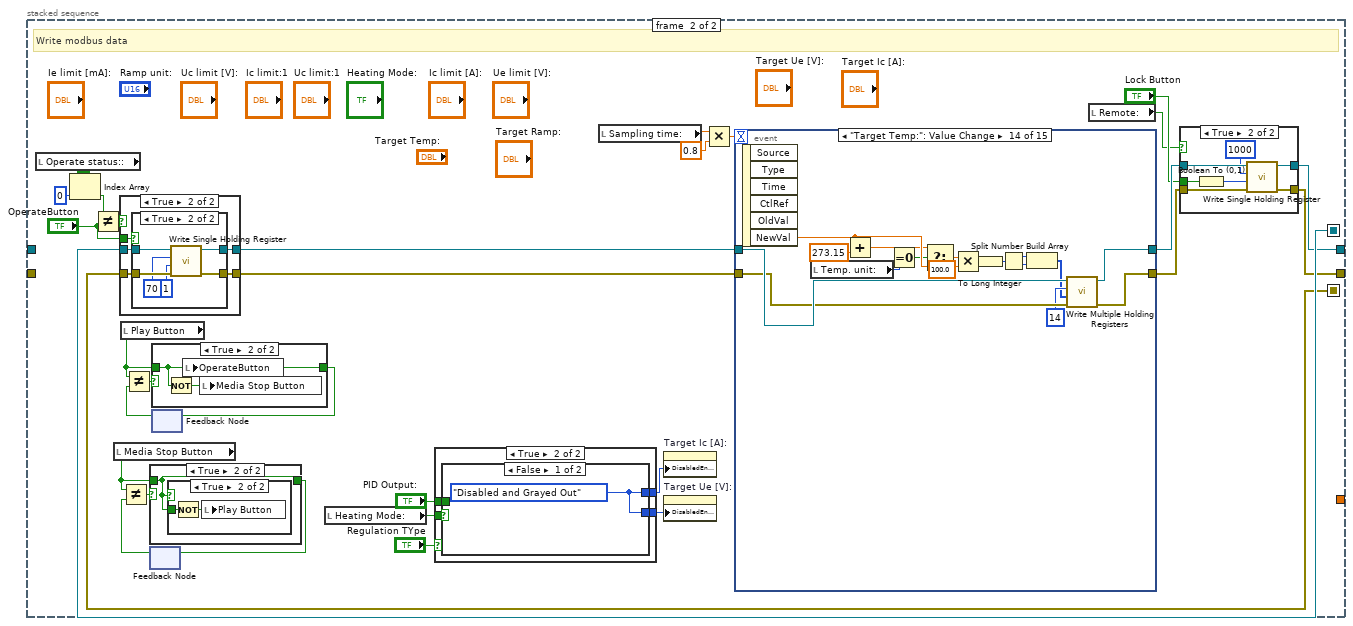
[diagram p16: hidden frame]
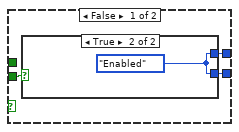
[diagram p18: hidden frame]
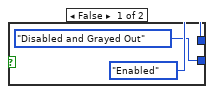
[diagram p19: hidden frame]
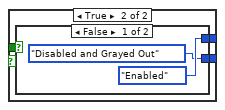
[diagram p20: hidden frame]
diagram:
  w13 = FALSE ("Connected:")
  n1 = case shown="False" TRUE {
    tunnel: [FALSE ("Visible") TRUE ("Visible")] -> w10
    tunnel: [FALSE ("Page Visible") TRUE ("Page Visible")] -> w4
    tunnel: [FALSE ("Visible") TRUE ("Visible")] -> w1
    frame False {
      # "Only HEAT3"
    }
    frame True {
      # "HEAT+TDS"
    }
  }
  n2 = control-ref of="Tab Control"() -> (w6:refnum<vi>)
  n3 = property class="TabCtl (strict)"(reference=w6) -> ("Pages"=w9:refnum<vi>[])  [unwired: 1 in, 2 out]
  n4 = Index Array(array=w9, index #1=1 ("index"), index #2=3 ("index")) -> (element #1=w7:refnum<vi>, element #2=w3:refnum<vi>)
  n5 = property on="Tab Control 3" class="TabCtl (strict)"("Visible"=w10) -> ()  [unwired: 2 in, 2 out]
  n6 = property class="Page"(reference=w7, "PageVis"=w4) -> ()  [unwired: 1 in, 2 out]
  n7 = property class="Page"(reference=w3, "PageVis"=w4) -> ()  [unwired: 1 in, 2 out]
  n8 = property on="Waveform Graph" class="WFGraph (strict)"("ActYScl"=1, "YScale.Visible"=w1) -> ()  [unwired: 2 in, 2 out]
  n9 = property on="PID manual setting" class="Tbl (strict)"("Index Values"=cluster{"Row":u32, "Column":u32} {"Row"=0, "Column"=0}) -> ()  [unwired: 2 in, 2 out]
  n10 = stacked-sequence {
    seq-local: [w103 _ _] -> [_ w163 _]
    seq-local: [w56 _ _] -> [_ w162 _]
    seq-local: [string[] ["OFF", "OFF"] ("Write Attribute") _ _] -> [_ w161 _]
    seq-local: [w121 _ _] -> [_ w160 _]
    seq-local: [dbl[][] [] _ _] -> [_ w142 _]
    seq-local: [T12 0 ("SRSRGA Refnum") _ _] -> [_ w149 _]
    seq-local: [errorcluster {"status"=FALSE, "code"=0, "source"=""} ("error out") _ _] -> [_ w148 _]
    seq-local: [w55 _ _] -> [_ w147 _]
    frame #0 {
      w27 = "HEAT3 Sampling time"  # Key 1
      w41 = "Recepice"  # Key 4
      w48 = "HEAT3 PID manual tab"  # Key 3
      w54 = "HEAT3 PID tab 1"  # Key 2
      w40 = "Section 2" ("section")
      w110 = "HEAT3 Path"  # Key 1
      w28 = "Section 1" ("section")
      w121 = string[] ["ON", "ON"] ("Write Attribute")
      w37 = FALSE ("Boolean")
      n11 = call <vilib>:"Dflt Data Dir.vi"() -> ("App:Default Data Directory"=w115:path)
      n12 = local write "Connected:"(w37) -> ()
      n13 = Build Path(base path=w115, name or relative path=path "TDS Configuration File.ini" ("default name")) -> ()  [unwired: 1 out]
      n14 = call <vilib>:"Application Directory.vi"() -> ("Application Directory"=w34:path)
      n15 = property on="Filament:" class="Bool"("Strings [4]"=w121) -> ()  [unwired: 2 in, 2 out]
      n16 = property on="CEM:" class="Bool"("Strings [4]"=w121) -> ()  [unwired: 2 in, 2 out]
      n17 = control-ref of="This VI"() -> (w120:refnum<vi>)
      n18 = Build Path(base path=w34, name or relative path="TDS Configuration File.ini") -> (appended path=w33:path)
      n19 = Get Date/Time In Seconds() -> (seconds since 1Jan1904=→"HEAT start time":timestamp)
      n20 = call-poly <vilib>:"Create Master Instance.vi"("address"="Address:") -> ("error out"=w104:errorcluster, "TCP master instance"=w105:refnum<class "Modbus Master.lvclass">)  [unwired: 9 in]
      n21 = property class="VI" props=["Front Panel.PanelBounds", "Front Panel.Resizeable"](reference=w120) -> (reference out=w118:refnum<vi>, error out=w117:errorcluster, "Front Panel.PanelBounds"=w119:T20)  [unwired: 1 in, 1 out]
      n22 = call-dynamic "Read Holding Registers.vi"("error in (no error)"=w104, "number of holding registers"=u16 100, "starting address"=u16 0, "Modbus master in"=w105) -> ("error out"=w56:errorcluster, "register values"=w98:u16[], "Modbus master out"=w103:refnum<class "Modbus Master.lvclass">)  [unwired: 5 in]
      n23 = case shown="No Error" w56 {
        tunnel: [0 5] -> w55
        tunnel: [T7."HEAT3 control" ("Tab Control 2") T7."HEAT3 configurations" ("Tab Control 2")] -> w20
        frame No Error {
        }
        frame Error {
        }
      }
      n24 = property on="main Graph" class="WFChart (strict)"("Visible"=w37) -> ()  [unwired: 2 in, 2 out]
      n25 = property class="VI"(reference=w118, error in=w117, "Front Panel.PanelBounds"=w119) -> ()  [unwired: 2 out]
      n26 = call <vilib>:"Open Config Data.vi"("create file if necessary (T)"=TRUE ("create file if necessary? (T)"), "configuration file path"=w33) -> ("error out"=w108:errorcluster, "refnum"=w109:T21)  [unwired: 7 in, 1 out]
      n27 = call-poly <vilib>:"Read Key.vi"("section"=w28, "error in (no error)"=w108, "key"=w110, "refnum"=w109) -> ("error out"=w24:errorcluster, "value"=w112:string, "found?"=w111:bool, "refnum out"=w26:T21)  [unwired: 2 in, 2 out]
      n28 = Index Array(array=w98, index #1=51 ("index"), index #2=52 ("index"), index #3=53 ("index"), index #4=54 ("index"), index #5=55 ("index"), index #6=56 ("index"), index #7=22 ("index"), index #8=21 ("index"), index #9=57 ("index"), index #10=58 ("index"), index #11=61 ("index"), index #12=44 ("index")) -> (element #1=w89:u16, element #2=w88:u16, element #3=w87:u16, element #4=w75:u16, element #5=w86:u16, element #6=w74:u16, element #7=w78:u16, element #8=w22:u16, element #9=w67:u16, element #10=w60:u16, element #11=w59:u16, element #12=w57:u16)
      n29 = case shown="True" w111 {
        tunnel: w112 -> [_ w140]
        frame False {
        }
        frame True {
          n30 = local write "Address:"(w140) -> ()
        }
      }
      n31 = Number To Fractional String(number=250.0) -> (F-format string=w31:string)  [unwired: 3 in]
      n32 = local write "Tab Control 2"(w20) -> ()
      n33 = local write "Tab Control"(T4."Main" ("Tab Control")) -> ()
      n34 = local write "Tab Control 3"(enum32{"RGA control", "RGA setting"}."RGA control" ("Tab Control 3")) -> ()
      n35 = call-poly <vilib>:"Read Key.vi"("section"=w28, "error in (no error)"=w24, "default value"=w31, "key"=w27, "refnum"=w26) -> ("error out"=w23:errorcluster, "value"=w30:string, "refnum out"=w25:T21)  [unwired: 1 in, 3 out]
      n36 = Divide(x=w89, y=100.0) -> (x/y=w85:dbl)
      n37 = Divide(x=w88, y=100.0) -> (x/y=w84:dbl)
      n38 = Divide(x=w87, y=100.0) -> (x/y=w83:dbl)
      n39 = Divide(x=w75, y=100.0) -> (x/y=w82:dbl)
      n40 = Divide(x=w86, y=10.0) -> (x/y=w81:dbl)
      n41 = Divide(x=w74, y=10.0) -> (x/y=w80:dbl)
      n42 = Not Equal To 0?(x=w78) -> (x != 0?=w77:bool)
      n43 = Not Equal To 0?(x=w22) -> (x != 0?=w71:bool)
      n44 = Not Equal To 0?(x=w67) -> (x != 0?=w70:bool)
      n45 = Divide(x=w60, y=100.0) -> (x/y=w64:dbl)
      n46 = Divide(x=w59, y=10.0) -> (x/y=w63:dbl)
      n47 = Fract/Exp String To Number(string=w30) -> (number=w29:dbl)  [unwired: 3 in, 1 out]
      n48 = local write "Ic limit:1"(w85) -> ()
      n49 = local write "Uc limit:1"(w84) -> ()
      n50 = local write "Ic limit [A]:"(w83) -> ()
      n51 = local write "Uc limit [V]:"(w82) -> ()
      n52 = local write "Ie limit [mA]:"(w81) -> ()
      n53 = local write "Ue limit [V]:"(w80) -> ()
      n54 = local write "Heating Mode:"(w77) -> ()
      n55 = local write "Regulation TYpe"(w71) -> ()
      n56 = local write "PID Output:"(w70) -> ()
      n57 = local write "Target Ic [A]:"(w64) -> ()
      n58 = local write "Target Ue [V]:"(w63) -> ()
      n59 = local write "Ramp unit:"(w57) -> ()
      n60 = local write "Sampling time:"(w29) -> ()
      n61 = call-poly <vilib>:"Read Key.vi"("section"=w40, "error in (no error)"=w23, "key"=w54, "refnum"=w25) -> ("error out"=w49:errorcluster, "value"=w52:string, "found?"=w53:bool, "refnum out"=w50:T21)  [unwired: 2 in, 2 out]
      n62 = case shown="True" w53 {
        tunnel: w52 -> [_ w135]
        frame False {
        }
        frame True {
          n63 = Spreadsheet String To Array(format string="%s", spreadsheet string=w135, array type (2D Dbl)=string[][] [] ("PID auto tab")) -> (array=w132:string[][])  [unwired: 1 in]
          n64 = local write "PID auto tab"(w132) -> ()
        }
      }
      n65 = call-poly <vilib>:"Read Key.vi"("section"=w40, "error in (no error)"=w49, "key"=w48, "refnum"=w50) -> ("error out"=w45:errorcluster, "value"=w46:string, "found?"=w47:bool, "refnum out"=w43:T21)  [unwired: 2 in, 2 out]
      n66 = case shown="True" w47 {
        tunnel: w46 -> [_ w129]
        frame False {
        }
        frame True {
          n67 = Spreadsheet String To Array(format string="%s", spreadsheet string=w129, array type (2D Dbl)=string[][] [] ("PID auto tab")) -> (array=w128:string[][])  [unwired: 1 in]
          n68 = local write "PID manual setting"(w128) -> ()
        }
      }
      n69 = call-poly <vilib>:"Read Key.vi"("section"=w40, "error in (no error)"=w45, "key"=w41, "refnum"=w43) -> ("error out"=w44:errorcluster, "value"=w38:string, "found?"=w39:bool, "refnum out"=w42:T21)  [unwired: 2 in, 2 out]
      n70 = case shown="True" w39 {
        tunnel: w38 -> [_ w127]
        frame False {
        }
        frame True {
          n71 = property on="XY Graph" class="XYGraph (strict)"() -> ("CrsrList"=w126:T22)  [unwired: 2 in, 2 out]
          n72 = Unflatten From String(type=w126, binary string=w127) -> (value=w125:T22)  [unwired: 3 in, 2 out]
          n73 = property on="XY Graph" class="XYGraph (strict)"("CrsrList"=w125) -> ()  [unwired: 2 in, 2 out]
        }
      }
      n74 = call <vilib>:"Close Config Data.vi"("error in (no error)"=w44, "write file if changed (T)"=FALSE ("write configuration file? (T)"), "refnum"=w42) -> ("error out"=w36:errorcluster)  [unwired: 8 out]
      n75 = call <vilib>:"Clear Errors.vi"("error in (no error)"=w36) -> ()  [unwired: 5 in, 2 out]
      "stopped_loops" <- w37
      "Boolean" <- w37
    }
    frame #1 {
      n76 = Initialize Array(0.0 ("element"), 20 ("dimension size")) -> (w144:dbl[])
      n77 = Tick Count (ms)() -> (millisecond timer value=w143:u32)
      n78 = while {
        tunnel: [TRUE] -> w152
        stop <- w1201 stop-if-true
        # "Recipe control"
        n79 = local read "Actual step:"() -> (w1191:i32)
        n80 = event shown="[0] Timeout" {
          selector: _ -> [_ _ _ _]
          dyn-events: _ -> [_ _ _ _]
          timeout: 250 -> [_ _ _ _]
          event Timeout {
            n81 = event-data() -> ()  [unwired: 1 in, 3 out]
          }
          event "Play Button": Value Change {
            w1254 = u16 1 items=["/s", "/m", "/h"] ("Ramp unit:")
            n82 = event-data() -> ()  [unwired: 1 in, 6 out]
            n83 = Get Date/Time In Seconds() -> (seconds since 1Jan1904=→"StartTime":timestamp)
            n84 = local write "Ramp unit:"(w1254) -> ()
          }
          event "Media Stop Button": Value Change {
            n85 = event-data() -> ()  [unwired: 1 in, 6 out]
            n86 = local read "output cluster"() -> (w1260:T3)
            n87 = Unbundle By Name(w1260) -> ("Time"=w1259:dbl[])
            n88 = Multiply(x=w1259, y=60.0) -> (x*y=w1258:dbl[])
            n89 = Get Date/Time In Seconds() -> (seconds since 1Jan1904=w1261:timestamp)
            n90 = Array Max & Min(array=w1258) -> (max value=w1257:dbl)  [unwired: 3 out]
            n91 = Subtract(x=w1261, y=w1257) -> (x-y=w1256:timestamp)
            n92 = local write "StartTime"(w1256) -> ()
          }
          event "ResetActRamp": Value Change {
            n93 = event-data() -> ("OldVal"=w1269:bool, "NewVal"=w1268:bool)  [unwired: 1 in, 4 out]
            n94 = Not(x=w1269) -> (.not. x?=w1267:bool)
            n95 = local read "OperateButton"() -> (w1266:bool)
            n96 = local read "Adv.RampControl"() -> (w1265:bool)
            n97 = And(x=w1267, y=w1268) -> (x .and. y?=w1264:bool)
            n98 = Compound Arithmetic op=AND(w1266, w1265, w1264) -> (w1263:bool)
            n99 = case shown="True" w1263 {
              frame False {
              }
              frame True {
                n100 = stacked-sequence {
                  frame #0 {
                    n101 = local write "OperateButton"(FALSE) -> ()
                  }
                  frame #1 {
                    n102 = Wait Until Next ms Multiple(millisecond multiple=u32 510) -> ()  [unwired: 1 out]
                  }
                  frame #2 {
                    n103 = local write "OperateButton"(TRUE) -> ()
                  }
                }
              }
            }
          }
        }
        n104 = case shown="1.." w1191 {
          tunnel: w1191 -> [_ w1241]
          frame ..0, Default {
          }
          frame 1.. {
            w1233 = 0.1 ("y")
            n105 = local read "output cluster"() -> (w1244:T3)
            n106 = local read "Target Ramp:"() -> (w1235:dbl)
            n107 = Unbundle By Name(w1244) -> ("Temp"=w1243:dbl[], "Ramp"=w1242:dbl[])
            n108 = local read "Target Temp:"() -> (w1240:dbl)
            n109 = Index Array(array=w1243, index=w1241) -> (element=w1239:dbl)
            n110 = Index Array(array=w1242, index=w1241) -> (element=w1237:dbl)
            n111 = Add(x=w1235, y=w1233) -> (x+y=w1236:dbl)
            n112 = Subtract(x=w1235, y=w1233) -> (x-y=w1234:dbl)
            n113 = Not Equal?(x=w1239, y=w1240) -> (x != y?=w1238:bool)
            n114 = In Range and Coerce(upper limit=w1236, x=w1237, lower limit=w1234) -> (In Range?=w1232:bool)  [unwired: 1 out]
            n115 = Not Equal?(x=w1237, y=w1235) -> ()  [unwired: 1 out]
            n116 = Not(x=w1232) -> (.not. x?=w1231:bool)
            n117 = case shown="True" w1238 {
              tunnel: w1239 -> [_ w1246]
              frame False {
              }
              frame True {
                n118 = property on="Target Temp:" class="DigNum (strict)"("Val(Sgnl)"=w1246) -> ()  [unwired: 2 in, 2 out]
              }
            }
            n119 = case shown="True" w1231 {
              tunnel: w1237 -> [_ w1245]
              frame False {
              }
              frame True {
                n120 = property on="Target Ramp:" class="DigNum (strict)"("Val(Sgnl)"=w1245) -> ()  [unwired: 2 in, 2 out]
              }
            }
          }
        }
        n121 = local read "output cluster"() -> (w1198:T3)
        n122 = local read "Boolean"() -> (w1201:T2)
        n123 = local read "StartTime"() -> (w1195:timestamp)
        n124 = Unbundle By Name(w1198) -> ("Time"=w1196:dbl[])
        n125 = Multiply(x=w1196, y=60.0) -> (x*y=w1194:dbl[])
        n126 = Add(x=w1195, y=w1194) -> (x+y=w1193:timestamp[])
        "x+y" <- w1193
        n127 = Get Date/Time In Seconds() -> (seconds since 1Jan1904=w1192:timestamp)
        n128 = for {
          tunnel: w1193 -> [w1248] mode=indexing
          tunnel: w1192 -> [w1249]
          tunnel: [w1250] -> w1190
          tunnel: [w1247] -> w1187
          i -> [w1252]
          stop <- w1253 stop-if-true
          n129 = Less?(x=w1249, y=w1248) -> (x < y?=w1253:bool)
          n130 = Subtract(x=w1249, y=w1248) -> (x-y=w1247:dbl)
          n131 = Select(t=w1252, s=w1253, f=0) -> (s? t:f=w1250:i32)
        }
        "Actual step:" <- w1190
        "Actual step:" <- w1190
        n132 = Not Equal To 0?(x=w1190) -> (x != 0?=w1186:bool)
        n133 = Not(x=w1186) -> (.not. x?=w1189:bool)
        n134 = local write "Play Button"(w1186) -> ()
        n135 = Select(t=w1187, s=w1186, f=0.0) -> (s? t:f=w1188:dbl)
        n136 = local write "Media Stop Button"(w1189) -> ()
        n137 = Absolute Value(x=w1188) -> (abs(x)=→"To next step [s]:":dbl)
        n138 = case shown="True" "Adv.RampControl" {
          frame False {
          }
          frame True {
            w1220 = 1.1 ("y")
            n139 = local read "Target Ramp:"() -> (w1210:dbl)
            n140 = local read "Act. Ramp:"() -> (w1221:dbl)
            n141 = local read "heat_LastData"() -> (w1216:dbl[])
            n142 = Multiply(x=w1210, y=w1220) -> (x*y=w1219:dbl)
            n143 = Divide(x=w1210, y=w1220) -> (x/y=w1218:dbl)
            n144 = Index Array(array=w1216, index #1=0 ("index (row)"), index #2=1 ("index (row)")) -> (element #1=w1213:dbl, element #2=w1211:dbl)
            n145 = In Range and Coerce(upper limit=w1219, x=w1221, lower limit=w1218) -> (In Range?=w1203:bool)  [unwired: 1 out]
            n146 = local read "Text Ring 3"() -> (w1208:u16)
            n147 = Multiply(x=10.0 ("y"), y=w1210) -> (x*y=w1207:dbl)
            n148 = case shown="0, Default" w1208 {
              tunnel: w1207 -> [w1223 w1226 w1229]
              tunnel: [w1223 w1224 w1227] -> w1205
              frame 0, Default {
              }
              frame 1 {
                n149 = Divide(x=w1226, y=60.0) -> (x/y=w1224:dbl)
              }
              frame 2 {
                w1228 = 60.0 ("y")
                n150 = Divide(x=w1229, y=w1228) -> (x/y=w1230:dbl)
                n151 = Divide(x=w1230, y=w1228) -> (x/y=w1227:dbl)
              }
            }
            n152 = Add(x=w1211, y=w1205) -> (x+y=w1212:dbl)
            n153 = Subtract(x=w1211, y=w1205) -> (x-y=w1217:dbl)
            n154 = In Range and Coerce(upper limit=w1212, x=w1213, lower limit=w1217) -> (In Range?=w1206:bool)  [unwired: 1 out]
            n155 = Not(x=w1206) -> (.not. x?=w1204:bool)
            n156 = And(x=w1204, y=w1203) -> (x .and. y?=w1202:bool)
            n157 = case shown="False" w1202 {
              tunnel: w1202 -> [_ w1222]
              frame False {
              }
              frame True {
                n158 = property on="ResetActRamp" class="Bool (strict)"("Val(Sgnl)"=w1222) -> ()  [unwired: 2 in, 2 out]
              }
            }
          }
        }
      }
      n159 = while {
        stop <- w684 stop-if-true
        (unwired) u32 500 ("millisecond multiple")
        # "Graf loop"
        n160 = case shown="True" "Start 2" {
          tunnel: "Sampling time:" -> [_ w686]
          frame False {
          }
          frame True {
            n161 = local read "Ie Act.:"() -> (w692:dbl)
            n162 = Multiply(x=w692, y=1000.0) -> (x*y=w694:dbl)
            n163 = local read "Uc Act.:"() -> (w689:dbl)
            n164 = local read "Ue Act.:"() -> (w690:dbl)
            n165 = local read "Ic Act.:"() -> (w691:dbl)
            n166 = Bundle(cluster=T6 {"[0]"=0.0, "[1]"=0.0, "[2]"=0.0, "[3]"=0.0}, "[0]"=w691, "[1]"=w694, "[2]"=w689, "[3]"=w690) -> (→"main Graph 2":T6)
            n167 = Divide(x=w686, y=1000.0) -> (x/y=w687:dbl)
            n168 = property on="main Graph 2" class="WFChart (strict)"("XScale.Multiplier"=w687) -> ()  [unwired: 2 in, 2 out]
          }
        }
        n169 = event shown="[9] \"Save As Button\": Value Change" {
          selector: _ -> [_ _ _ _ _ _ _ _ _ _ _ _ _]
          dyn-events: _ -> [_ _ _ _ _ _ _ _ _ _ _ _ _]
          timeout: 1 -> [_ _ _ _ _ _ _ _ _ _ _ _ _]
          tunnel: [_ w791 _ w802 _ _ _ _ _ _ _ _ _] -> w684
          tunnel: T15 {"Name"="0", "Color"=16776960, "Style"=4, "Point Style"=3, "Name Visible"=FALSE, "Allow Drag"=TRUE, "Cursor Mode"=0, "Plot"=0, "Index"=0, "Position"={"X"=0.0, "Y"=0.0}, "X Scale"=0, "Y Scale"=0, "Watch Plots"=[], "Watch All Plots"=FALSE, "Plot Area"=0, "Label Offset"={"X"=1.0408340855860843e-17, "Y"=0.5847953216374269}} ("element") -> [_ _ _ _ w807 w852 w877 _ _ _ _ w936 _]
          event Timeout {
            # "Axies name:"
            n170 = event-data() -> ()  [unwired: 1 in, 3 out]
            n171 = property on="Temp. unit:" class="Ring (strict)"() -> ("RingText.Text"=w716:string)  [unwired: 2 in, 2 out]
            n172 = local read "Actual step:"() -> (w727:i32)
            n173 = property on="Units:" class="Enum (strict)"() -> ("RingText.Text"=w722:string)  [unwired: 2 in, 2 out]
            n174 = local read "Act. Temp:"() -> (w733:dbl)
            n175 = property on="XY Graph" class="XYGraph (strict)"() -> ("CrsrList"=w732:T22)  [unwired: 2 in, 2 out]
            n176 = feedback #1() -> (w725:dbl)  [unwired: 1 in]
            n177 = Equal To 0?(x=w727) -> (x = 0?=w728:bool)
            n178 = Concatenate Strings("Temperature [" ("string"), w716, "]" ("string")) -> (w715:string)
            n179 = Concatenate Strings("Pressure [" ("string"), w722, "]" ("string")) -> (w719:string)
            n180 = case shown="True" w728 {
              tunnel: w733 -> [_ w763]
              tunnel: w732 -> [w757 w765]
              tunnel: [w756 w764] -> w731
              tunnel: [w758 w763] -> w726
              tunnel: w725 -> [w758 _]
              frame False {
                n181 = Index Array(array=w757, index=0) -> (element=w761:T15)
                n182 = Bundle By Name(cluster=w761, "Position.Y"=w758) -> (w760:T15)
                n183 = Replace Array Subset(array=w757, new element=w760, index=0) -> (w756:T22)
              }
              frame True {
                n184 = Index Array(array=w765, index=0) -> (element=w768:T15)
                n185 = Bundle By Name(cluster=w768, "Position.Y"=w763) -> (w767:T15)
                n186 = Replace Array Subset(array=w765, new element=w767, index=0) -> (w764:T22)
              }
            }
            n187 = feedback-in #1(w726) -> ()
            n188 = property on="Waveform Graph" class="WFGraph (strict)"("ActYScl"=0, "YScale.NameLbl.Text"=w715, "ActYScl"=1, "YScale.NameLbl.Text"=w719) -> ()  [unwired: 2 in, 2 out]
            n189 = local read "Specifications"() -> (w714:T9)
            n190 = for {
              tunnel: w731 -> [w782] mode=indexing
              tunnel: [w778] -> w738 mode=indexing
              tunnel: [w776] -> w737 mode=indexing
              tunnel: [w781] -> w734 mode=indexing
              shift-right: [w778] -> _
              shift-left: _ -> [w779]
              shift-right: [w776] -> _
              shift-left: _ -> [w777]
              tunnel: [w771] -> w730 mode=indexing
              i -> [w780]
              n191 = Unbundle By Name(w782) -> ("Position"=w781:cluster{"X":dbl, "Y":dbl}, "Position.X"=w778:dbl, "Position.Y"=w776:dbl)
              n192 = case shown="1, Default" w780 {
                tunnel: [w783 0.0] -> w772
                tunnel: w779 -> [w789 _]
                tunnel: w778 -> [w788 _]
                tunnel: w777 -> [w787 _]
                tunnel: w776 -> [w786 _]
                frame 1, Default {
                  n193 = Subtract(x=w788, y=w789) -> (x-y=w784:dbl)
                  n194 = Subtract(x=w786, y=w787) -> (x-y=w785:dbl)
                  n195 = Divide(x=w785, y=w784) -> (x/y=w783:dbl)
                }
                frame 0 {
                }
              }
              n196 = Absolute Value(x=w772) -> (abs(x)=w775:dbl)
              n197 = Less?(x=w775, y=0.1) -> (x < y?=w773:bool)
              n198 = Select(t="Default Ramp:", s=w773, f=w772) -> (s? t:f=w771:dbl)
            }
            "Temperature_Pos_Tab" <- w734
            n199 = for {
              tunnel: w714 -> [w755] mode=indexing
              tunnel: [w747] -> w711
              i -> [w754]
              stop <- w746 stop-if-true
              n200 = Unbundle By Name(w755) -> ("Mass"=w751:i32)
              n201 = Number To Decimal String(number=w751) -> (decimal integer string=w750:string)  [unwired: 1 in]
              n202 = Add(x=w754, y=2) -> (x+y=w747:i32)
              n203 = Concatenate Strings("Mass: " ("string"), w750) -> (w749:string)
              n204 = property on="Waveform Graph" class="WFGraph (strict)"("Active Plot"=w747, "Plot.Plot Name"=w749, "Plot.Visible?"=TRUE, "Plot.YScaleIdx"=1) -> (error out=w746:errorcluster)  [unwired: 2 in, 1 out]
            }
            n205 = Subtract(x=20, y=w711) -> (x-y=w712:i32)
            n206 = local write "XY Graph"(w734) -> ()
            n207 = for {
              N: w712 -> [_]
              tunnel: w711 -> [w743]
              i -> [w744]
              stop <- w739 stop-if-true
              n208 = Increment(x=w744) -> (x+1=w742:i32)
              n209 = Add(x=w743, y=w742) -> (x+y=w741:i32)
              n210 = property on="Waveform Graph" class="WFGraph (strict)"("Active Plot"=w741, "Plot.Visible?"=FALSE) -> (error out=w739:errorcluster)  [unwired: 2 in, 1 out]
            }
            n211 = Absolute Value(x=w730) -> (abs(x)=w729:dbl[])
            n212 = Bundle By Name(cluster=T3 {"Time"=[], "Temp"=[], "Ramp"=[]}, "Time"=w738, "Temp"=w737, "Ramp"=w729) -> (→"output cluster":T3)
          }
          event Panel Close {
            w791 = TRUE
            n213 = event-data() -> ()  [unwired: 1 in, 4 out]
            n214 = while {
              tunnel: w791 -> [w793]
              stop <- w794 stop-if-true
              n215 = local write "Boolean"(w793) -> ()
              n216 = local read "stopped_loops"() -> (w794:bool)
              n217 = Wait (ms)(milliseconds to wait=10) -> ()  [unwired: 1 out]
            }
          }
          event "Temp. unit:": Value Change {
            n218 = event-data() -> ()  [unwired: 1 in, 6 out]
            n219 = property on="Temp. unit:" class="Ring (strict)"() -> ("Strings []"=w799:string[], "Value"=w797:u16)  [unwired: 2 in, 2 out]
            n220 = Reverse 1D Array(array=w799) -> (reversed array=w798:string[])
            n221 = Index Array(array=w798, index=w797) -> (element=w796:string)
            n222 = Concatenate Strings("Temperature [" ("string"), w796, "]" ("string")) -> (w795:string)
            n223 = property on="main Graph" class="WFChart (strict)"("YScale.NameLbl.Text"=w795) -> ()  [unwired: 2 in, 2 out]
            n224 = property on="XY Graph" class="XYGraph (strict)"("YScale.NameLbl.Text"=w795) -> ()  [unwired: 2 in, 2 out]
          }
          event "stop": Value Change {
            w802 = TRUE
            n225 = event-data() -> ()  [unwired: 1 in, 6 out]
            n226 = while {
              tunnel: w802 -> [w803]
              stop <- w805 stop-if-true
              n227 = local write "Boolean"(w803) -> ()
              n228 = Wait (ms)(milliseconds to wait=10) -> ()  [unwired: 1 out]
              n229 = local read "stopped_loops"() -> (w805:bool)
            }
          }
          event "XY Graph": Mouse Up {
            n230 = event-data() -> ("Mods.Double Click"=w806:bool, "Coords"=w808:T23)  [unwired: 1 in, 6 out]
            n231 = case shown="True" w806 {
              tunnel: w808 -> [_ w828]
              tunnel: w807 -> [_ w821]
              frame False {
              }
              frame True {
                n232 = property on="XY Graph" class="XYGraph (strict)"() -> ("Plot Area:Size"=w844:T24, "Plot Area:Position"=w845:T25, "X Scale.Range"=w843:T26, "Y Scale.Range"=w842:T26, "Old Cursor List"=w827:T27)  [unwired: 2 in, 2 out]
                n233 = Unbundle By Name(w828) -> ("Horizontal"=w813:i32, "Vertical"=w812:i32)
                n234 = Unbundle By Name(w844) -> ("Width"=w814:u32, "Height"=w811:u32)
                n235 = Unbundle By Name(w845) -> ("Left"=w810:i32, "Top"=w809:i32)
                n236 = Unbundle By Name(w843) -> ("Maximum"=w839:dbl, "Minimum"=w838:dbl)
                n237 = Unbundle By Name(w842) -> ("Maximum"=w841:dbl, "Minimum"=w840:dbl)
                n238 = Index Array(array=w827) -> (element=w826:T28)  [unwired: 1 in]
                n239 = Unbundle By Name(w826) -> ("Position"=w825:cluster{"X":dbl, "Y":dbl})
                n240 = Subtract(x=w839, y=w838) -> (x-y=w834:dbl)
                n241 = Subtract(x=w841, y=w840) -> (x-y=w833:dbl)
                n242 = Add(x=w810, y=w814) -> (x+y=w819:u32)
                n243 = Add(x=w811, y=w809) -> (x+y=w818:u32)
                n244 = In Range and Coerce(upper limit=w819, x=w813, lower limit=w810) -> (In Range?=w816:bool)  [unwired: 1 out]
                n245 = In Range and Coerce(upper limit=w818, x=w812, lower limit=w809) -> (In Range?=w817:bool)  [unwired: 1 out]
                n246 = And(x=w816, y=w817) -> (x .and. y?=w815:bool)
                n247 = property on="XY Graph" class="XYGraph (strict)"() -> ("CrsrList"=w820:T22)  [unwired: 2 in, 2 out]
                n248 = Subtract(x=w812, y=w809) -> (x-y=w832:i32)
                n249 = Subtract(x=w813, y=w810) -> (x-y=w837:i32)
                n250 = Divide(x=w834, y=w814) -> (x/y=w836:dbl)
                n251 = Subtract(x=w811, y=w832) -> (x-y=w831:u32)
                n252 = Divide(x=w833, y=w811) -> (x/y=w835:dbl)
                n253 = Multiply(x=w836, y=w837) -> (x*y=w830:dbl)
                n254 = Array Size(array=w820) -> (size(s)=w824:i32)
                n255 = Multiply(x=w835, y=w831) -> (x*y=w829:dbl)
                n256 = Bundle By Name(cluster=w825, "X"=w830, "Y"=w829) -> (w822:cluster{"X":dbl, "Y":dbl})
                n257 = Number To Decimal String(number=w824) -> (decimal integer string=w823:string)  [unwired: 1 in]
                n258 = case shown="True" w815 {
                  tunnel: w823 -> [_ w851]
                  tunnel: w822 -> [_ w850]
                  tunnel: w821 -> [_ w849]
                  tunnel: w820 -> [_ w848]
                  frame False {
                  }
                  frame True {
                    n259 = Bundle By Name(cluster=w849, "Name"=w851, "Position"=w850) -> (w847:T15)
                    n260 = Insert Into Array(array=w848, new element=w847) -> (w846:T22)  [unwired: 1 in]
                    n261 = property on="XY Graph" class="XYGraph (strict)"("CrsrList"=w846) -> ()  [unwired: 2 in, 2 out]
                  }
                }
              }
            }
          }
          event "Add Step": Value Change {
            n262 = event-data() -> ()  [unwired: 1 in, 5 out]
            n263 = property on="XY Graph" class="XYGraph (strict)"() -> ("CrsrList"=w871:T22)  [unwired: 2 in, 2 out]
            n264 = Array Size(array=w871) -> (size(s)=w856:i32)
            n265 = Decrement(x=w856) -> (x-1=w870:i32)
            n266 = Index Array(array=w871, index=w870) -> (element=w869:T15)
            n267 = Unbundle By Name(w869) -> ("Position"=w858:cluster{"X":dbl, "Y":dbl})
            n268 = Unbundle By Name(w858) -> ("X"=w860:dbl, "Y"=w859:dbl)
            n269 = Add(x=w859, y=10.0) -> (x+y=w866:dbl)
            n270 = Add(x=w859, y=10.0) -> (x+y=w861:dbl)
            n271 = Add(x=2.0, y=w860) -> (x+y=w867:dbl)
            n272 = Add(x=4.0, y=w860) -> (x+y=w862:dbl)
            n273 = Bundle By Name(cluster=w858, "X"=w867, "Y"=w866) -> (w874:cluster{"X":dbl, "Y":dbl})
            n274 = Bundle By Name(cluster=w858, "X"=w862, "Y"=w861) -> (w857:cluster{"X":dbl, "Y":dbl})
            n275 = Increment(x=w856) -> (x+1=w855:i32)
            n276 = Number To Decimal String(number=w856) -> (decimal integer string=w875:string)  [unwired: 1 in]
            n277 = Number To Decimal String(number=w855) -> (decimal integer string=w854:string)  [unwired: 1 in]
            n278 = Bundle By Name(cluster=w852, "Name"=w875, "Position"=w874) -> (w873:T15)
            n279 = Bundle By Name(cluster=w852, "Name"=w854, "Position"=w857) -> (w853:T15)
            n280 = Insert Into Array(array=w871, new element #1=w873, new element #2=w853) -> (w872:T22)  [unwired: 1 in]
            n281 = property on="XY Graph" class="XYGraph (strict)"("CrsrList"=w872) -> ()  [unwired: 2 in, 2 out]
          }
          event "Remove": Value Change {
            n282 = event-data() -> ()  [unwired: 1 in, 6 out]
            n283 = Build Array(w877) -> (w876:T29)
            n284 = property on="XY Graph" class="XYGraph (strict)"("CrsrList"=w876) -> ()  [unwired: 2 in, 2 out]
          }
          event "Remove STEP": Value Change {
            w878 = 2 ("x")
            n285 = event-data() -> ()  [unwired: 1 in, 6 out]
            n286 = property on="XY Graph" class="XYGraph (strict)"() -> ("CrsrList"=w883:T22)  [unwired: 2 in, 2 out]
            n287 = Array Size(array=w883) -> (size(s)=w879:i32)
            "size(s) 2" <- w879
            n288 = Subtract(x=w879, y=w878) -> (x-y=w882:i32)
            n289 = Delete From Array(array=w883, length=w878, index=w882) -> (array with subset deleted=w881:T22)  [unwired: 1 out]
            n290 = Array Size(array=w881) -> (size(s)=→"size(s)":i32)
            n291 = property on="XY Graph" class="XYGraph (strict)"("CrsrList"=w881) -> ()  [unwired: 2 in, 2 out]
          }
          event "Clear ALL": Value Change {
            n292 = event-data() -> ()  [unwired: 1 in, 6 out]
            n293 = property on="main Graph" class="WFChart (strict)"("History Data"=T16 []) -> ()  [unwired: 2 in, 2 out]
          }
          event "Save As Button": Value Change {
            w896 = T30 2 items=["User Home"=0, "User Desktop"=1, "User Documents"=2, "User Application Data"=3, "User Preferences"=4, "User Temporary"=5, "Public Documents"=6, "Public Application Data"=7, "Public Preferences"=8, "Public Cache"=13, "System Core Libraries"=9, "System Installed Libraries"=10, "Application Files"=11, "Boot Volume Root"=12] ("system directory type")
            n294 = event-data() -> ()  [unwired: 1 in, 6 out]
            n295 = local read "Waveform Graph"() -> (w889:waveform(dbl)[])
            n296 = Get Date/Time In Seconds() -> (seconds since 1Jan1904=w894:timestamp)
            n297 = Format Date/Time String() -> ()  [unwired: 3 in, 1 out]
            n298 = Format Date/Time String(time format string (%c)="%H.%M.%S", seconds (now)=w894) -> (date/time string=w893:string)  [unwired: 1 in]
            n299 = call <vilib>:"Get System Directory.vi"("create directory if not found? (F)"=TRUE, "system directory type"=w896) -> ("system directory"=w895:path)  [unwired: 9 in]
            n300 = Concatenate Strings("TDS_" ("default name"), w893, ".txt" ("default name")) -> (w891:string)
            n301 = call "File Dialog"("start path"=w895, "default name"=w891) -> ("selected path"=w885:path, "error out"=w887:errorcluster)  [unwired: 10 in, 2 out]
            n302 = call-poly <vilib>:"Export Waveforms to Spreadsheet File.vi"("error in (no error)"=w887, "waveforms"=w889, "file path (dialog if empty)"=w885) -> ("error out"=w890:errorcluster)  [unwired: 7 in, 1 out]
            n303 = call <vilib>:"Clear Errors.vi"("error in (no error)"=w890) -> ()  [unwired: 5 in, 2 out]
          }
          event "Saveproject": Value Change {
            n304 = event-data() -> ()  [unwired: 1 in, 6 out]
            n305 = property on="XY Graph" class="XYGraph (strict)"() -> ("CrsrList"=w909:T22)  [unwired: 2 in, 2 out]
            n306 = local read "Regulation TYpe"() -> (w906:bool)
            n307 = local read "Heating Mode:"() -> (w903:bool)
            n308 = local read "Specifications"() -> (w910:T9)
            n309 = local read "Target Ue [V]:"() -> (w905:dbl)
            n310 = local read "Target Ramp:"() -> (w898:dbl)
            n311 = local read "Target Temp:"() -> (w899:dbl)
            n312 = local read "Target Ic [A]:"() -> (w904:dbl)
            n313 = for {
              tunnel: w909 -> [w916] mode=indexing
              tunnel: [w915] -> w908 mode=indexing
              n314 = Unbundle By Name(w916) -> ("Position"=w915:cluster{"X":dbl, "Y":dbl})
            }
            n315 = local read "PID Output:"() -> (w907:bool)
            n316 = local read "Temp. unit:"() -> (w901:u16)
            n317 = local read "Ramp unit:"() -> (w900:u16)
            n318 = Bundle By Name(cluster="TDS", "Target Temp:"=w899, "Target Ramp:"=w898, "Ramp unit:"=w900, "Temp. unit:"=w901, "Target Ue [V]:"=w905, "Target Ic [A]:"=w904, "Heating Mode:"=w903, "PID Output:"=w907, "Regulation Type"=w906, "RGA Specifications"=w910, "Heating Recipe"=w908) -> (w902:T1)
            n319 = call "File Dialog2"("default name"="TDS_ProcessConfig.json") -> ("selected path"=w913:path, "cancelled"=w912:bool)  [unwired: 11 in, 2 out]
            n320 = case shown="False" w912 {
              tunnel: w913 -> [w917 _]
              tunnel: w902 -> [w929 _]
              frame False {
                w918 = TRUE ("replace all? (F)")
                n321 = Flatten To JSON(anything=w929) -> (JSON string=w925:string, 11:w926:errorcluster)  [unwired: 2 in]
                n322 = Search and Replace String(replace all?=w918, input string=w925, search string="},{", replace string="},\n{" ("search string"), error in=w926) -> (result string=w924:string, error out=w920:errorcluster)  [unwired: 3 in, 2 out]
                n323 = Search and Replace String(replace all?=w918, input string=w924, search string=",\"", replace string=",\n    \"" ("search string"), error in=w920) -> (result string=w921:string, error out=w919:errorcluster)  [unwired: 3 in, 2 out]
                n324 = Open/Create/Replace File(file path (use dialog)=w917, error in=w919, operation (0:open)=T17."replace or create with confirmation") -> (refnum out=w934:refnum<file>, error out=w933:errorcluster)  [unwired: 3 in, 1 out]
                n325 = Write to Text File(file (use dialog)=w934, text=w921, error in=w933) -> (refnum out=w932:refnum<file>, error out=w931:errorcluster)  [unwired: 1 in, 1 out]
                n326 = Close File(refnum=w932, error in=w931) -> (error out=w930:errorcluster)  [unwired: 1 out]
                n327 = call <vilib>:"Clear Errors.vi"("error in (no error)"=w930) -> ()  [unwired: 5 in, 2 out]
              }
              frame True {
              }
            }
          }
          event "Loadproject": Value Change {
            n328 = event-data() -> ()  [unwired: 1 in, 6 out]
            n329 = call "File Dialog3"("default name"="TDS_ProcessConfig.json") -> ("selected path"=w939:path, "exists"=w937:bool, "cancelled"=w938:bool)  [unwired: 11 in, 1 out]
            n330 = case shown="False" w938 {
              tunnel: w939 -> [w942 _]
              tunnel: w937 -> [w943 _]
              tunnel: w936 -> [w941 _]
              frame False {
                n331 = case shown="True" w943 {
                  tunnel: w942 -> [_ w959]
                  tunnel: w941 -> [_ w953]
                  frame False {
                  }
                  frame True {
                    n332 = Open/Create/Replace File(file path (use dialog)=w959, operation (0:open)=T17."open") -> (refnum out=w965:refnum<file>, error out=w964:errorcluster)  [unwired: 4 in, 1 out]
                    n333 = Read from Text File(file (use dialog)=w965, error in=w964) -> (refnum out=w960:refnum<file>, text=w963:string, error out=w961:errorcluster)  [unwired: 2 in, 1 out]
                    n334 = Unflatten From JSON(JSON string=w963, type and defaults="TDS 2", error in (no error)=w961) -> (value=w957:T1, error out=w962:errorcluster)  [unwired: 4 in]
                    n335 = Unbundle By Name(w957) -> ("Target Temp:"=w951:dbl, "Target Ramp:"=w950:dbl, "Ramp unit:"=w949:u16, "Temp. unit:"=w956:u16, "Target Ue [V]:"=w948:dbl, "Target Ic [A]:"=w947:dbl, "Heating Mode:"=w946:bool, "PID Output:"=w945:bool, "Regulation Type"=w944:bool, "RGA Specifications"=w955:T9, "Heating Recipe"=w952:cluster{"X":dbl, "Y":dbl}[])
                    n336 = for {
                      tunnel: [w972] -> w954 mode=indexing
                      tunnel: w953 -> [w971]
                      tunnel: w952 -> [w970] mode=indexing
                      i -> [w969]
                      n337 = Number To Decimal String(number=w969) -> (decimal integer string=w968:string)  [unwired: 1 in]
                      n338 = Bundle By Name(cluster=w971, "Position"=w970, "Name"=w968) -> (w972:T15)
                    }
                    n339 = local write "Specifications"(w955) -> ()
                    n340 = Close File(refnum=w960, error in=w962) -> (error out=w966:errorcluster)  [unwired: 1 out]
                    n341 = local write "Temp. unit:"(w956) -> ()
                    n342 = call <vilib>:"Clear Errors.vi"("error in (no error)"=w966) -> ()  [unwired: 5 in, 2 out]
                    n343 = property on="Target Ramp:" class="DigNum (strict)"("Val(Sgnl)"=w950) -> ()  [unwired: 2 in, 2 out]
                    n344 = property on="Target Ic [A]:" class="DigNum (strict)"("Val(Sgnl)"=w947) -> ()  [unwired: 2 in, 2 out]
                    n345 = property on="PID Output:" class="Bool (strict)"("Val(Sgnl)"=w945) -> ()  [unwired: 2 in, 2 out]
                    n346 = property on="Target Temp:" class="DigNum (strict)"("Val(Sgnl)"=w951) -> ()  [unwired: 2 in, 2 out]
                    n347 = property on="Ramp unit:" class="Ring (strict)"("Val(Sgnl)"=w949) -> ()  [unwired: 2 in, 2 out]
                    n348 = property on="Target Ue [V]:" class="DigNum (strict)"("Val(Sgnl)"=w948) -> ()  [unwired: 2 in, 2 out]
                    n349 = property on="Heating Mode:" class="Bool (strict)"("Val(Sgnl)"=w946) -> ()  [unwired: 2 in, 2 out]
                    n350 = property on="Regulation TYpe" class="Bool (strict)"("Val(Sgnl)"=w944) -> ()  [unwired: 2 in, 2 out]
                    n351 = property on="XY Graph" class="XYGraph (strict)"("CrsrList"=w954) -> ()  [unwired: 2 in, 2 out]
                  }
                }
              }
              frame True {
              }
            }
          }
          event "Clear ALL 2": Value Change {
            n352 = event-data() -> ()  [unwired: 1 in, 6 out]
            n353 = property on="main Graph 2" class="WFChart (strict)"("History Data"=T18 []) -> ()  [unwired: 2 in, 2 out]
          }
        }
        n354 = Wait Until Next ms Multiple(millisecond multiple="Sampling time:") -> ()  [unwired: 1 out]
        n355 = case shown="True" "Start 1" {
          frame False {
          }
          frame True {
            (unwired) 0.5 ("y")
            n356 = Get Date/Time In Seconds() -> (seconds since 1Jan1904=w701:timestamp)
            n357 = local read "Sampling time:"() -> (w699:dbl)
            n358 = property on="main Graph" class="WFChart (strict)"() -> ("History Data"=w704:T16)  [unwired: 2 in, 2 out]
            n359 = for {
              tunnel: w704 -> [w710] mode=indexing
              tunnel: [w709] -> w703 mode=indexing
              n360 = Cluster To Array(cluster=w710) -> (array=w709:dbl[])
            }
            n361 = Divide(x=w699, y=1000.0) -> (x/y=w698:dbl)
            n362 = Transpose 2D Array(2D array=w703) -> (transposed array=w702:dbl[][])
            n363 = for {
              tunnel: w701 -> [w708]
              tunnel: w698 -> [w707]
              tunnel: w702 -> [w706] mode=indexing
              tunnel: [w705] -> w700 mode=indexing
              n364 = Bundle By Name("Y"=w706, "dt"=w707, "t0"=w708) -> (w705:waveform(dbl))  [unwired: 1 out]
            }
            "Waveform Graph" <- w700
          }
        }
        n365 = local read "heat_LastData"() -> (w677:dbl[])
        n366 = local read "RGA_LastData"() -> (w678:sgl[])
        n367 = Insert Into Array(array=w677, new element=w678) -> (w679:dbl[])  [unwired: 1 in]
        n368 = Array To Cluster(array=w679) -> (cluster=→"main Graph":T5)
      }
      n369 = while {
        tunnel: [TRUE] -> w150
        shift-right: [w991] -> w165
        shift-left: w149 -> [w990]
        shift-right: [w978] -> w164
        shift-left: w148 -> [w989]
        tunnel: w161 -> [w984]
        tunnel: w160 -> [w983]
        i -> [w974]
        stop <- w988 stop-if-true
        # "RGA loop"
        n370 = local read "Connected:"() -> (w981:bool)
        n371 = event shown="[5] \"START RGA\", \"START RGA  2\": Value Change" {
          selector: _ -> [_ _ _ _ _ _ _ _ _]
          dyn-events: _ -> [_ _ _ _ _ _ _ _ _]
          timeout: 250 -> [_ _ _ _ _ _ _ _ _]
          tunnel: [w1007 w1035 w1052 w1066 w1087 w1117 w1163 w1173 T12 0 ("SRSRGA Refnum")] -> w991
          tunnel: w990 -> [w1008 w1037 w1055 w1072 w1092 w1119 _ w1170 w1182]
          tunnel: w989 -> [w1006 w1036 w1054 w1071 w1091 w1118 _ w1169 w1181]
          tunnel: [w996 w1034 w1053 w1070 w1090 w1116 w1162 w1172 w1179] -> w978
          tunnel: w984 -> [w1004 w1032 w1050 _ _ _ _ _ _]
          tunnel: w983 -> [w1003 w1031 w1049 _ _ _ _ _ _]
          tunnel: "Electron Emission [mA]" -> [_ w1028 _ w1069 _ _ _ _ _]
          tunnel: [w997 T14."Enabled" ("Disabled") _ _ _ T14."Disabled and Grayed Out" ("Disabled") _ _ _] -> w976
          tunnel: [T14."Disabled and Grayed Out" ("Disabled") T14."Disabled and Grayed Out" ("Disabled") _ _ _ T14."Enabled" ("Disabled") _ _ _] -> w975
          event Timeout {
            n372 = event-data() -> ()  [unwired: 1 in, 3 out]
            n373 = local read "Connected:"() -> (w1005:bool)
            n374 = local read "CEM:"() -> (w1000:bool)
            n375 = case shown="True" w1005 {
              tunnel: w1008 -> [w1013 w1016]
              tunnel: [w1013 w1024] -> w1007
              tunnel: w1006 -> [w1011 w1021]
              tunnel: [w1011 w1014] -> w996
              tunnel: [T14."Disabled and Grayed Out" ("Disabled") T14."Enabled" ("Disabled")] -> w997
              frame False {
              }
              frame True {
                n376 = call "SRSRGAo Set or Query CEM Status.vi"("error in (no error)"=w1021, "CEM (Unchanged)"=enum16{"Unchanged", "Off", "On"}."Unchanged", "SRSRGA Refnum"=w1016) -> ("error out"=w1015:errorcluster, "CEM On?"=w1019:bool, "SRSRGA Refnum"=w1022:T12)  [unwired: 6 in]
                n377 = local write "CEM:"(w1019) -> ()
                n378 = call "SRSRGAo Set or Query Electron Emission.vi"("error in (no error)"=w1015, "Electron Emission (1.00 mA)"=sgl -1.0, "SRSRGA Refnum"=w1022) -> ("error out"=w1014:errorcluster, "Electron Emission"=w1018:sgl, "SRSRGA Refnum"=w1024:T12)  [unwired: 6 in]
                "Act. Electron Emission" <- w1018
                n379 = Not Equal To 0?(x=w1018) -> (x != 0?=w1023:bool)
                n380 = local write "Filament:"(w1023) -> ()
              }
            }
            n381 = local read "Filament:"() -> (w1002:bool)
            n382 = Select(t=w1004, s=w1000, f=w1003) -> (s? t:f=w999:string[])
            n383 = property on="CEM:" class="Bool"("Strings [4]"=w999) -> ()  [unwired: 2 in, 2 out]
            n384 = Select(t=w1004, s=w1002, f=w1003) -> (s? t:f=w1001:string[])
            n385 = property on="Filament:" class="Bool"("Strings [4]"=w1001) -> ()  [unwired: 2 in, 2 out]
            n386 = property on="Filament:" class="Bool"("DisabledEnum"=w997) -> ()  [unwired: 2 in, 2 out]
            n387 = property on="CEM:" class="Bool"("DisabledEnum"=w997) -> ()  [unwired: 2 in, 2 out]
            n388 = disable-structure shown="Enabled" {
              disable-tunnel: w996 -> [w1009 _]
              frame Disabled {
                n389 = case shown="Error" w1009 {
                  frame No Error {
                  }
                  frame Error {
                    n390 = property on="Reconnect" class="Bool (strict)"("Val(Sgnl)"=TRUE ("Value (Signaling)")) -> ()  [unwired: 2 in, 2 out]
                  }
                }
              }
              frame Enabled {
              }
            }
          }
          event "Filament:": Value Change {
            n391 = event-data() -> ()  [unwired: 1 in, 6 out]
            n392 = local read "Filament:"() -> (w1033:bool)
            n393 = property on="Filament:" class="Bool"("DisabledEnum"=u8 2 ("Write Attribute")) -> ()  [unwired: 2 in, 2 out]
            n394 = Not(x=w1033) -> (.not. x?=w1039:bool)
            n395 = Select(t=w1028, s=w1039, f=sgl 0.0) -> (s? t:f=w1042:sgl)
            n396 = Select(t=w1032, s=w1039, f=w1031) -> (s? t:f=w1038:string[])
            n397 = call "SRSRGAo Set or Query Electron Emission.vi"("error in (no error)"=w1036, "Electron Emission (1.00 mA)"=w1042, "SRSRGA Refnum"=w1037) -> ("error out"=w1034:errorcluster, "SRSRGA Refnum"=w1035:T12)  [unwired: 6 in, 1 out]
            n398 = call "SRSRGA Error Handler.vi"("error in (no error)"=w1034) -> ("error?"=w1040:bool)  [unwired: 9 in, 1 out]
            n399 = case shown="False" w1040 {
              tunnel: w1039 -> [w1044 _]
              tunnel: [u8 0 ("Write Attribute") u8 0 ("Write Attribute")] -> w1029
              tunnel: w1038 -> [w1043 _]
              frame False {
                n400 = property on="Filament:" class="Bool"("Strings [4]"=w1043) -> ()  [unwired: 2 in, 2 out]
                n401 = local write "Filament:"(w1044) -> ()
              }
              frame True {
              }
            }
            n402 = property on="Filament:" class="Bool"("DisabledEnum"=w1029) -> ()  [unwired: 2 in, 2 out]
          }
          event "CEM:": Value Change {
            n403 = event-data() -> ()  [unwired: 1 in, 6 out]
            n404 = local read "CEM:"() -> (w1051:bool)
            n405 = property on="CEM:" class="Bool"("DisabledEnum"=u8 2 ("Write Attribute")) -> ()  [unwired: 2 in, 2 out]
            n406 = Not(x=w1051) -> (.not. x?=w1059:bool)
            n407 = Select(t=w1050, s=w1059, f=w1049) -> (s? t:f=w1060:string[])
            n408 = Select(t=enum16{"Unchanged", "Off", "On"}."On" ("CEM (Unchanged)"), s=w1059, f=enum16{"Unchanged", "Off", "On"}."Off" ("CEM (Unchanged)")) -> (s? t:f=w1058:enum16{"Unchanged", "Off", "On"})
            n409 = call "SRSRGAo Set or Query CEM Status.vi"("error in (no error)"=w1054, "CEM (Unchanged)"=w1058, "SRSRGA Refnum"=w1055) -> ("error out"=w1053:errorcluster, "SRSRGA Refnum"=w1052:T12)  [unwired: 6 in, 1 out]
            n410 = call "SRSRGA Error Handler.vi"("error in (no error)"=w1053) -> ("error?"=w1061:bool)  [unwired: 9 in, 1 out]
            n411 = case shown="False" w1061 {
              tunnel: w1059 -> [w1062 _]
              tunnel: [u8 0 ("Write Attribute") u8 0 ("Write Attribute")] -> w1047
              tunnel: w1060 -> [w1063 _]
              frame False {
                n412 = property on="CEM:" class="Bool"("Strings [4]"=w1063) -> ()  [unwired: 2 in, 2 out]
                n413 = local write "CEM:"(w1062) -> ()
              }
              frame True {
              }
            }
            n414 = property on="CEM:" class="Bool"("DisabledEnum"=w1047) -> ()  [unwired: 2 in, 2 out]
          }
          event "ionizer": Value Change {
            n415 = event-data() -> ()  [unwired: 1 in, 6 out]
            n416 = local read "Filament:"() -> (w1073:bool)
            n417 = call "SRSRGAo Get Session.vi"("SRSRGA Refnum"=w1072) -> ("SRSRGA Session"=w1075:refnum<visa-resource-name>)
            n418 = property class="Instr"(reference=w1075, "Timeout"=u32 300000 ("General Settings:Timeout Value")) -> ()  [unwired: 1 in, 2 out]
            n419 = call "SRSRGAa Ionizer Dialog.vi"("error in (no error)"=w1071, "Emission On?"=w1073, "Electron Emission (0.02-3.50 mA)"=w1069, "SRSRGA Refnum"=w1072) -> ("error out"=w1076:errorcluster, "Electron Emission"=w1068:sgl, "SRSRGA Refnum"=w1067:T12)  [unwired: 5 in]
            n420 = local write "Electron Emission [mA]"(w1068) -> ()
            n421 = Unbundle By Name(w1076) -> ("code"=w1079:i32)
            n422 = Greater Or Equal?(x=w1079, y=5000) -> (x >= y?=w1077:bool)
            n423 = case shown="True" w1077 {
              tunnel: w1076 -> [w1081 w1085]
              tunnel: [w1081 w1084] -> w1070
              tunnel: w1067 -> [w1080 w1082]
              tunnel: [w1080 w1082] -> w1066
              frame False {
              }
              frame True {
                n424 = call "SRSRGAo Get Session.vi"("SRSRGA Refnum"=w1082) -> ("SRSRGA Session"=w1083:refnum<visa-resource-name>)
                n425 = call "SRSRGAc IN Initialize.vi"("error in (no error)"=w1085, "Initialization Level"=T19."Initialize", "SRSRGA Session"=w1083) -> ("error out"=w1084:errorcluster)  [unwired: 5 in, 3 out]
              }
            }
            n426 = call "SRSRGA Error Handler.vi"("error in (no error)"=w1070) -> ()  [unwired: 9 in, 2 out]
          }
          event "detector": Value Change {
            n427 = event-data() -> ()  [unwired: 1 in, 6 out]
            n428 = call "SRSRGAo Get Session.vi"("SRSRGA Refnum"=w1092) -> ("SRSRGA Session"=w1094:refnum<visa-resource-name>)
            n429 = property class="Instr"(reference=w1094, "Timeout"=u32 300000 ("General Settings:Timeout Value")) -> ()  [unwired: 1 in, 2 out]
            n430 = local read "CEM:"() -> (w1089:bool)
            n431 = call "SRSRGAa Detector Dialog.vi"("error in (no error)"=w1091, "CEM On?"=w1089, "SRSRGA Refnum"=w1092) -> ("error out"=w1095:errorcluster, "SRSRGA Refnum"=w1088:T12)  [unwired: 7 in]
            n432 = Unbundle By Name(w1095) -> ("code"=w1098:i32)
            n433 = Greater Or Equal?(x=w1098, y=5000) -> (x >= y?=w1096:bool)
            n434 = case shown="True" w1096 {
              tunnel: w1095 -> [w1100 w1103]
              tunnel: [w1100 w1102] -> w1090
              tunnel: w1088 -> [w1099 w1101]
              tunnel: [w1099 w1101] -> w1087
              frame False {
              }
              frame True {
                n435 = call "SRSRGAo Get Session.vi"("SRSRGA Refnum"=w1101) -> ("SRSRGA Session"=w1104:refnum<visa-resource-name>)
                n436 = call "SRSRGAc IN Initialize.vi"("error in (no error)"=w1103, "Initialization Level"=T19."Initialize", "SRSRGA Session"=w1104) -> ("error out"=w1102:errorcluster)  [unwired: 5 in, 3 out]
              }
            }
            n437 = call "SRSRGA Error Handler.vi"("error in (no error)"=w1090) -> ()  [unwired: 9 in, 2 out]
          }
          event "START RGA", "START RGA  2": Value Change {
            w1109 = T14."Disabled and Grayed Out" ("Disabled")
            w1108 = T14."Enabled" ("Disabled")
            w1113 = u8 2 ("Write Attribute")
            n438 = event-data() -> ()  [unwired: 1 in, 6 out]
            n439 = property on="Filament:" class="Bool"("DisabledEnum"=w1113) -> ()  [unwired: 2 in, 2 out]
            n440 = call "SRSRGAo Start Table Scan.vi"("error in (no error)"=w1118, "Specifications"="Specifications", "SRSRGA Refnum"=w1119) -> ("error out"=w1129:errorcluster, "CEM On?"=w1127:bool, "Specifications"=w1106:T31, "SRSRGA Refnum"=w1128:T12, "Noise Floor"=w1126:i32)  [unwired: 4 in]
            n441 = for {
              tunnel: [w1130] -> _ mode=indexing
              tunnel: [w1131] -> w1107
              tunnel: w1106 -> [w1130] mode=indexing
              stop <- w1131 stop-if-true
              n442 = Unbundle By Name(w1130) -> ("CEM On?"=w1131:bool)
            }
            n443 = property on="P vs. t" class="WFChart (strict)"("History Data"=sgl[][] [] ("Write Attribute"), "X Scale.Offset and Multiplier:Multiplier"="Rate (sec)") -> ()  [unwired: 2 in, 2 out]
            n444 = property on="CEM:" class="Bool"("DisabledEnum"=w1113) -> ()  [unwired: 2 in, 2 out]
            n445 = property on="stop 4" class="Bool"("DisabledEnum"=w1108) -> ()  [unwired: 2 in, 2 out]
            n446 = property on="START RGA  2" class="Bool"("DisabledEnum"=w1109) -> ()  [unwired: 2 in, 2 out]
            n447 = Multiply(x=1000, y="Rate (sec)") -> (x*y=w1122:dbl)
            n448 = property on="stop 3" class="Bool"("DisabledEnum"=w1108) -> ()  [unwired: 2 in, 2 out]
            n449 = property on="START RGA" class="Bool"("DisabledEnum"=w1109) -> ()  [unwired: 2 in, 2 out]
            n450 = local write "CEM:"(w1107) -> ()
            n451 = while {
              tunnel: w1122 -> [w1141]
              tunnel: [w1138] -> w1115
              tunnel: "Units:" -> [w1132]
              shift-left: w1126 -> [w1150]
              shift-right: [w1133] -> _
              tunnel: [w1137] -> w1114
              shift-left: w1127 -> [w1152]
              shift-right: [w1151] -> _
              tunnel: w1106 -> [w1135]
              tunnel: w1128 -> [w1153]
              tunnel: w1129 -> [w1154]
              shift-right: [w1142] -> _
              shift-left: _ -> [w1144]
              tunnel: [u8 0 ("Write Attribute")] -> w1112
              stop <- w1147 continue-if-true
              n452 = Wait Until Next ms Multiple(millisecond multiple=w1141) -> ()  [unwired: 1 out]
              n453 = call "SRSRGAo Measure Table.vi"("Entrance Noise Floor"=w1150, "Units"=w1132, "error in (no error)"=w1154, "Entrance CEM On?"=w1152, "Specifications"=w1135, "SRSRGA Refnum"=w1153) -> ("error out"=w1137:errorcluster, "Exit CEM On?"=w1151:bool, "Readings in Units"=w1139:sgl[], "SRSRGA Refnum"=w1138:T12, "Exit Noise Floor"=w1133:i32)  [unwired: 1 in]
              "RGA_LastData" <- w1139
              n454 = local write "Filament:"(TRUE ("Filament")) -> ()
              n455 = Tick Count (ms)() -> (millisecond timer value=w1142:u32)
              n456 = Subtract(x=w1142, y=w1144) -> (x-y=→"Loop Time [ms]":u32)
              n457 = Reshape Array(w1139, 1 ("Dimension Size"), 4 ("Dimension Size")) -> (→"P vs. t" →"output array":sgl[][])
              n458 = stacked-sequence {
                tunnel: [w1159] -> w1148
                tunnel: w1133 -> [_]
                frame #0 {
                  n459 = local read "Boolean"() -> (w1158:T2)
                  n460 = Or(x="stop 4", y="stop 3") -> (x .or. y?=w1155:bool)
                  n461 = Or(x=w1155, y=w1158) -> (x .or. y?=w1159:T2)
                }
              }
              n462 = Unbundle By Name(w1137) -> ("status"=w1149:bool)
              n463 = Not Or(1:w1148, 2:w1149) -> (0:w1147:T2)
            }
            n464 = call "SRSRGAo Stop Table Scan.vi"("error in (no error)"=w1114, "SRSRGA Refnum"=w1115) -> ("error out"=w1116:errorcluster, "SRSRGA Refnum"=w1117:T12)  [unwired: 8 in]
            n465 = property on="CEM:" class="Bool"("DisabledEnum"=w1112) -> ()  [unwired: 2 in, 2 out]
            n466 = property on="Filament:" class="Bool"("DisabledEnum"=w1112) -> ()  [unwired: 2 in, 2 out]
          }
          event "Connect": Value Change {
            n467 = event-data() -> ()  [unwired: 1 in, 6 out]
            n468 = local read "Connection Type:"() -> (w1164:u16)
            n469 = call "SRSRGAo Open.vi"("Reinitialize? (True)"=TRUE ("Reinitialize? (False)"), "Connection Type"=w1164) -> ("error out"=w1162:errorcluster, "SRSRGA Refnum"=w1163:T12)  [unwired: 4 in, 4 out]
            n470 = case shown="No Error" w1162 {
              tunnel: [TRUE FALSE] -> w1161
              frame No Error {
              }
              frame Error {
              }
            }
            n471 = local write "Connected:"(w1161) -> ()
            n472 = local write "Reconnect"(FALSE ("Reconnect")) -> ()
          }
          event "Reconnect": Value Change {
            n473 = event-data() -> ()  [unwired: 1 in, 6 out]
            n474 = call "SRSRGAo Close.vi"("error in (no error)"=w1169, "SRSRGA Refnum"=w1170) -> ()  [unwired: 9 in, 1 out]
            n475 = local read "Connection Type:"() -> (w1174:u16)
            n476 = call "SRSRGAo Open.vi"("Reinitialize? (True)"=TRUE ("Reinitialize? (False)"), "Connection Type"=w1174) -> ("error out"=w1172:errorcluster, "SRSRGA Refnum"=w1173:T12)  [unwired: 4 in, 4 out]
            n477 = case shown="Error" w1172 {
              tunnel: [TRUE FALSE] -> w1171
              frame No Error {
              }
              frame Error {
              }
            }
            n478 = local write "Connected:"(w1171) -> ()
            n479 = local write "Reconnect"(FALSE ("Reconnect")) -> ()
          }
          event "Disconnect": Value Change {
            n480 = event-data() -> ()  [unwired: 1 in, 6 out]
            n481 = call "SRSRGAo Close.vi"("error in (no error)"=w1181, "SRSRGA Refnum"=w1182) -> ("error out"=w1179:errorcluster)  [unwired: 9 in]
            n482 = local write "Connected:"(FALSE) -> ()
          }
        }
        "Error out:" <- w978
        n483 = case shown="True" w981 {
          tunnel: [T14."Enabled" ("Disabled") T14."Disabled and Grayed Out" ("Disabled")] -> w980
          tunnel: [T14."Disabled and Grayed Out" ("Disabled") T14."Enabled" ("Disabled")] -> w979
          frame False {
          }
          frame True {
          }
        }
        n484 = property on="Disconnect" class="Bool"("DisabledEnum"=w979) -> ()  [unwired: 2 in, 2 out]
        n485 = property on="Connect" class="Bool"("DisabledEnum"=w980) -> ()  [unwired: 2 in, 2 out]
        n486 = property on="P vs. t" class="WFChart (strict)"() -> ("Plot.Plot Name"=→"Label.Text":string)  [unwired: 2 in, 2 out]
        n487 = Unbundle By Name(w978) -> ("status"=→"Error:":bool)
        n488 = local read "Boolean"() -> (w988:T2)
        n489 = property on="START RGA" class="Bool"("DisabledEnum"=w976) -> ()  [unwired: 2 in, 2 out]
        n490 = property on="START RGA  2" class="Bool"("DisabledEnum"=w976) -> ()  [unwired: 2 in, 2 out]
        n491 = property on="stop 3" class="Bool"("DisabledEnum"=w975) -> ()  [unwired: 2 in, 2 out]
        n492 = property on="stop 4" class="Bool"("DisabledEnum"=w975) -> ()  [unwired: 2 in, 2 out]
        "Numeric" <- w974
      }
      n493 = while {
        tunnel: [TRUE] -> w151
        shift-right: [w216] -> w155
        shift-left: w162 -> [w209]
        shift-right: [w219] -> w156
        shift-left: w163 -> [w218]
        shift-right: [w213] -> _
        shift-left: w143 -> [w212]
        shift-right: [w202] -> _
        shift-left: w147 -> [w207]
        tunnel: w142 -> [w214]
        shift-right: [w198] -> _
        shift-left: w144 -> [w201]
        stop <- w232 stop-if-true
        (unwired) u32 500 ("millisecond multiple")
        # "HEAT and PID cntrl"
        n494 = Tick Count (ms)() -> (millisecond timer value=w213:u32)
        n495 = event shown="[3] \"Reconect\": Value Change" {
          selector: _ -> [_ _ _ _]
          dyn-events: _ -> [_ _ _ _]
          timeout: 1 -> [_ _ _ _]
          tunnel: w214 -> [w616 _ _ _]
          tunnel: [w614 dbl[][] [] _ _] -> _
          tunnel: [w613 w619 errorcluster {"status"=TRUE, "code"=0, "source"="Connect to\nnew IP addres"} ("error constant") errorcluster {"status"=TRUE, "code"=0, "source"="Rconnecting"} ("error constant")] -> w208
          tunnel: w209 -> [w613 w619 _ _]
          tunnel: [w612 w618 0 0] -> w206
          tunnel: w207 -> [w612 w618 _ _]
          event Timeout {
            n496 = event-data() -> ()  [unwired: 1 in, 1 out]
            n497 = Select(t=w616, s=FALSE ("build array of data?"), f=dbl[][] []) -> (s? t:f=w614:dbl[][])
          }
          event "clean": Value Change {
            n498 = event-data() -> ()  [unwired: 1 in, 1 out]
            n499 = Get Date/Time In Seconds() -> (seconds since 1Jan1904=w620:timestamp)
            n500 = local write "HEAT start time"(w620) -> ()
            n501 = local write "clean"(FALSE ("clc graph")) -> ()
          }
          event "Address:": Value Change {
            n502 = event-data() -> ()  [unwired: 1 in, 1 out]
          }
          event "Reconect": Value Change {
            w625 = FALSE ("Connected:")
            n503 = event-data() -> ()  [unwired: 1 in, 1 out]
            n504 = local write "Comunication error:"(w625) -> ()
            n505 = local write "Connected:"(w625) -> ()
          }
        }
        n506 = Subtract(x=w213, y=w212) -> (x-y=→"Loop time:":u32)
        n507 = case shown="Error" w208 {
          selector: w208 -> [w632 w641]
          tunnel: [w632 w638] -> w204
          tunnel: w218 -> [w631 w640]
          tunnel: [w631 w639] -> w217
          tunnel: w206 -> [_ w636]
          tunnel: [0 w635] -> w202
          frame No Error {
            w628 = FALSE
            n508 = Not(x=w628) -> (.not. x?=w629:bool)
            n509 = local write "Comunication error:"(w628) -> ()
            n510 = local write "Connected:"(w629) -> ()
          }
          frame Error {
            n511 = Increment(x=w636) -> (x+1=w635:i32)
            n512 = Less?(x=w635, y=2) -> (x < y?=w634:bool)
            n513 = local write "Comunication error:"(TRUE) -> ()
            n514 = case shown="True" w634 {
              tunnel: w641 -> [w642 w650]
              tunnel: w640 -> [w643 w649]
              tunnel: [w643 w647] -> w639
              tunnel: [w642 w646] -> w638
              frame False {
              }
              frame True {
                n515 = call-dynamic "Close.vi"("error in (no error)"=w650, "Modbus master in"=w649) -> ("error out"=w645:errorcluster)  [unwired: 9 in]
                n516 = call <vilib>:"Clear Errors.vi"("error in (no error)"=w645) -> ("error out"=w644:errorcluster)  [unwired: 5 in, 1 out]
                n517 = local read "Address:"() -> (w648:string)
                n518 = call-poly <vilib>:"Create Master Instance.vi"("error in (no error)"=w644, "address"=w648) -> ("error out"=w646:errorcluster, "TCP master instance"=w647:refnum<class "Modbus Master.lvclass">)  [unwired: 8 in]
              }
            }
          }
        }
        "error out" <- w204
        n519 = Unbundle By Name(w204) -> ("status"=w205:bool)
        n520 = local read "Sampling time:"() -> (w188:dbl)
        n521 = Not(x=w205) -> (.not. x?=w203:bool)
        n522 = local write "Connected:"(w203) -> ()
        n523 = Wait Until Next ms Multiple(millisecond multiple=w188) -> ()  [unwired: 1 out]
        n524 = local read "Act. Temp:"() -> (w220:dbl)
        n525 = stacked-sequence {
          seq-local: [w261 _] -> [_ w341]
          seq-local: [w260 _] -> [_ w340]
          tunnel: w217 -> [w259 _]
          tunnel: w204 -> [w258 _]
          tunnel: [_ w333] -> w219
          tunnel: [_ w331] -> w216
          tunnel: [w249 _] -> w187
          frame #0 {
            # "read modbus data"
            n526 = call-dynamic "Read Holding Registers.vi"("error in (no error)"=w258, "number of holding registers"=u16 1, "starting address"=u16 1151, "Modbus master in"=w259) -> ("error out"=w256:errorcluster, "register values"=w250:u16[], "Modbus master out"=w257:refnum<class "Modbus Master.lvclass">)  [unwired: 5 in]
            n527 = Index Array(array=w250) -> (element=w251:u16)  [unwired: 1 in]
            n528 = Not Equal To 0?(x=w251) -> (x != 0?=w252:bool)
            "Remote:" <- w252
            n529 = case shown="False" w252 {
              tunnel: [T14."Disabled and Grayed Out" ("Disabled") T14."Enabled" ("Disabled")] -> w253
              frame False {
                n530 = local write "Lock Button"(FALSE ("Lock Button")) -> ()
              }
              frame True {
              }
            }
            n531 = local read "Act. Setpoint:"() -> (w274:dbl)
            n532 = disable-structure shown="Disabled" {
              disable-tunnel: [w304 u16 2] -> w279
              frame Disabled {
                n533 = Decrement(x="Channel:") -> (x-1=w304:u16)
              }
              frame Enabled {
              }
            }
            n534 = local read "Act. Temp:"() -> (w249:dbl)
            n535 = call-dynamic "Read Holding Registers.vi"("error in (no error)"=w256, "number of holding registers"=u16 1, "starting address"=u16 0, "Modbus master in"=w257) -> ("error out"=w292:errorcluster, "register values"=w267:u16[], "Modbus master out"=w293:refnum<class "Modbus Master.lvclass">)  [unwired: 5 in]
            n536 = property on="Lock Button" class="Bool (strict)"("DisabledEnum"=w253) -> ()  [unwired: 2 in, 2 out]
            n537 = call-dynamic "Read Holding Registers.vi"("error in (no error)"=w292, "number of holding registers"=u16 2, "starting address"=w279, "Modbus master in"=w293) -> ("error out"=w298:errorcluster, "register values"=w277:u16[], "Modbus master out"=w299:refnum<class "Modbus Master.lvclass">)  [unwired: 5 in]
            n538 = call "Modbus_Get_Status_list.vi"("register values"=w267) -> ("Boolean"=w271:bool, "Boolean 2"=→"Operate:":bool, "Boolean array"=→"Operate status::":bool[])  [unwired: 8 in]
            n539 = Build Array(w249, w274) -> (→"heat_LastData":dbl[])
            n540 = Not(x=w271) -> (.not. x?=→"Interlock:":bool)
            n541 = local read "New D:"() -> (w288:dbl)
            n542 = local read "New P:"() -> (w286:dbl)
            n543 = local read "New I:"() -> (w290:dbl)
            n544 = call-dynamic "Read Holding Registers.vi"("error in (no error)"=w298, "number of holding registers"=u16 3, "starting address"=u16 45, "Modbus master in"=w299) -> ("error out"=w281:errorcluster, "register values"=w269:u16[], "Modbus master out"=w283:refnum<class "Modbus Master.lvclass">)  [unwired: 5 in]
            n545 = call "Modbus_Pid_Control.vi"("register values"=w269, "new D"=w288, "new I"=w290, "new P"=w286) -> ("Numeric"=→"Act. D":dbl, "Numeric 2"=→"Act. I":dbl, "Numeric 3"=→"Act. P":dbl, "Boolean"=w268:bool)  [unwired: 4 in]
            "New PID request" <- w268
            n546 = call-dynamic "Read Holding Registers.vi"("error in (no error)"=w281, "number of holding registers"=u16 100, "starting address"=u16 0, "Modbus master in"=w283) -> ("error out"=w280:errorcluster, "register values"=w262:u16[], "Modbus master out"=w282:refnum<class "Modbus Master.lvclass">)  [unwired: 5 in]
            n547 = local read "Temp. unit:"() -> (w276:u16)
            n548 = case shown="True" w268 {
              tunnel: w282 -> [w307 w312]
              tunnel: w280 -> [w308 w311]
              tunnel: [w307 w310] -> w261
              tunnel: [w308 w309] -> w260
              frame False {
              }
              frame True {
                n549 = local read "New P:"() -> (w320:dbl)
                n550 = local read "New D:"() -> (w322:dbl)
                n551 = local read "New I:"() -> (w321:dbl)
                n552 = Multiply(x=w320, y=10.0) -> (x*y=w316:dbl)
                n553 = To Word Integer(number=w316) -> (16bit integer=w317:i16)
                n554 = To Word Integer(number=w321) -> (16bit integer=w318:i16)
                n555 = To Word Integer(number=w322) -> (16bit integer=w319:i16)
                n556 = Build Array(w317, w318, w319) -> (w313:i16[])
                n557 = call-dynamic "Write Multiple Holding Registers.vi"("error in (no error)"=w311, "holding register values"=w313, "starting address"=u16 45, "Modbus master in"=w312) -> ("error out"=w309:errorcluster, "Modbus master out"=w310:refnum<class "Modbus Master.lvclass">)  [unwired: 6 in]
              }
            }
            n558 = Index Array(array=w262, index=22) -> (element=w265:u16)
            n559 = call "Modbus_Get_Temp.vi"("register values"=w277, "Temp. unit:"="Temp. unit:") -> ("Numeric"=→"Act. Temp:":dbl, "Strings []"=w246:string[])  [unwired: 8 in]
            n560 = Not Equal To 0?(x=w265) -> (x != 0?=w264:bool)
            "EB active:" <- w264
            n561 = property on="Text Ring 3" class="Ring (strict)"("Strings []"=w246) -> ()  [unwired: 2 in, 2 out]
            n562 = call "Modbus_Decode_Multiple_registers.vi"("Temp. unit:"=w276, "register values"=w262) -> ("Numeric 3"=→"Uc Act.:" →"Uc Act.:" →"Uc Act.: 2":dbl, "Numeric 4"=→"Ic Act.:" →"Ic Act.:" →"Ic Act.: 2":dbl, "Numeric 5"=→"Act. Setpoint:":dbl, "Numeric 2"=→"Ie Act.:" →"Ie Act.: 2":dbl, "register"=→"Text Ring 3" →"Text Ring 4":u16, "Numeric"=→"Ue Act.:" →"Ue Act.: 2":dbl)  [unwired: 4 in]
            n563 = Not(x=w264) -> (.not. x?=→"RES active:":bool)
            n564 = property on="Text Ring 5" class="Ring (strict)"("Strings []"=w246) -> ()  [unwired: 2 in, 2 out]
            "Text Ring" <- "Temp. unit:"
            "Text Ring 2" <- "Temp. unit:"
            "Text Ring 6" <- "Temp. unit:"
          }
          frame #1 {
            # "Write modbus data"
            n565 = local read "Operate status::"() -> (w346:bool[])
            n566 = Index Array(array=w346, index=0) -> (element=w344:bool)
            n567 = Not Equal?(x=w344, y="OperateButton") -> (x != y?=w343:bool)
            n568 = local read "Media Stop Button"() -> (w323:bool)
            n569 = case shown="True" w343 {
              tunnel: w341 -> [w587 w592]
              tunnel: w340 -> [w586 w591]
              tunnel: [w587 w590] -> w325
              tunnel: [w586 w589] -> w324
              tunnel: "OperateButton" -> [_ w588]
              frame False {
              }
              frame True {
                n570 = case shown="True" w588 {
                  tunnel: w592 -> [w596 w604]
                  tunnel: w591 -> [w595 w603]
                  tunnel: [w594 w602] -> w590
                  tunnel: [w593 w601] -> w589
                  frame False {
                    n571 = call-dynamic "Write Single Holding Register.vi"("error in (no error)"=w595, "holding register value"=u16 1, "address"=u16 71, "Modbus master in"=w596) -> ("error out"=w593:errorcluster, "Modbus master out"=w594:refnum<class "Modbus Master.lvclass">)  [unwired: 6 in]
                  }
                  frame True {
                    n572 = call-dynamic "Write Single Holding Register.vi"("error in (no error)"=w603, "holding register value"=u16 1, "address"=u16 70, "Modbus master in"=w604) -> ("error out"=w601:errorcluster, "Modbus master out"=w602:refnum<class "Modbus Master.lvclass">)  [unwired: 6 in]
                  }
                }
              }
            }
            n573 = local read "Play Button"() -> (w352:bool)
            n574 = feedback #2() -> (w347:bool)  [unwired: 1 in]
            n575 = Not Equal?(x=w323, y=w347) -> (x != y?=w349:bool)
            n576 = case shown="True" w349 {
              tunnel: w323 -> [w605 w606]
              tunnel: [w605 w606] -> w348
              frame False {
              }
              frame True {
                n577 = case shown="True" w606 {
                  tunnel: w606 -> [_ w608]
                  frame False {
                  }
                  frame True {
                    n578 = Not(x=w608) -> (.not. x?=w607:bool)
                    n579 = local write "Play Button"(w607) -> ()
                  }
                }
              }
            }
            n580 = feedback-in #2(w348) -> ()
            n581 = feedback #3() -> (w350:bool)  [unwired: 1 in]
            n582 = Not Equal?(x=w352, y=w350) -> (x != y?=w353:bool)
            n583 = case shown="True" w353 {
              tunnel: w352 -> [w609 w611]
              tunnel: [w609 w611] -> w351
              frame False {
              }
              frame True {
                n584 = Not(x=w611) -> (.not. x?=w610:bool)
                n585 = local write "OperateButton"(w611) -> ()
                n586 = local write "Media Stop Button"(w610) -> ()
              }
            }
            n587 = feedback-in #3(w351) -> ()
            n588 = local read "Heating Mode:"() -> (w336:bool)
            n589 = case shown="True" "Regulation TYpe" {
              tunnel: [w364 w372] -> w338
              tunnel: [w363 w371] -> w337
              tunnel: w336 -> [w365 w370]
              tunnel: "PID Output:" -> [_ w369]
              frame False {
                n590 = case shown="True" w365 {
                  tunnel: [T14."Enabled" ("Disabled") w368] -> w364
                  tunnel: [T14."Disabled and Grayed Out" ("Disabled") w368] -> w363
                  frame False {
                  }
                  frame True {
                    w368 = T14."Enabled" ("Disabled")
                  }
                }
              }
              frame True {
                n591 = case shown="False" w370 {
                  tunnel: [w373 w375] -> w372
                  tunnel: [w373 w374] -> w371
                  tunnel: w369 -> [_ w376]
                  frame False {
                    w373 = T14."Disabled and Grayed Out" ("Disabled")
                  }
                  frame True {
                    n592 = case shown="False" w376 {
                      tunnel: [T14."Enabled" ("Disabled") T14."Disabled and Grayed Out" ("Disabled")] -> w375
                      tunnel: [T14."Disabled and Grayed Out" ("Disabled") T14."Enabled" ("Disabled")] -> w374
                      frame False {
                      }
                      frame True {
                      }
                    }
                  }
                }
              }
            }
            n593 = local read "Sampling time:"() -> (w328:dbl)
            n594 = property on="Target Ic [A]:" class="DigNum (strict)"("DisabledEnum"=w338) -> ()  [unwired: 2 in, 2 out]
            n595 = property on="Target Ue [V]:" class="DigNum (strict)"("DisabledEnum"=w337) -> ()  [unwired: 2 in, 2 out]
            n596 = Multiply(x=w328, y=0.8) -> (x*y=w326:dbl)
            n597 = event shown="[13] \"Target Temp:\": Value Change" {
              selector: _ -> [_ _ _ _ _ _ _ _ _ _ _ _ _ _ _]
              dyn-events: _ -> [_ _ _ _ _ _ _ _ _ _ _ _ _ _ _]
              timeout: w326 -> [_ _ _ _ _ _ _ _ _ _ _ _ _ _ _]
              tunnel: w325 -> [w384 w459 w468 w477 w486 w495 w504 w513 w522 w531 w539 w547 w555 w574 w582]
              tunnel: [w382 w460 w469 w478 w487 w496 w505 w514 w523 w532 w540 w548 w556 w571 w583] -> w332
              tunnel: w324 -> [w381 w458 w467 w476 w485 w494 w503 w512 w521 w530 w538 w546 w554 w573 w581]
              tunnel: [w383 w461 w470 w479 w488 w497 w506 w515 w524 w533 w541 w549 w557 w572 w584] -> w334
              event Timeout {
                n598 = event-data() -> ()  [unwired: 1 in, 3 out]
                n599 = case shown="No Error" w381 {
                  tunnel: w384 -> [w435 w456]
                  tunnel: w381 -> [w434 w455]
                  tunnel: [w433 w456] -> w383
                  tunnel: [w432 w455] -> w382
                  frame No Error {
                    n600 = call-dynamic "Read Holding Registers.vi"("error in (no error)"=w434, "number of holding registers"=u16 100, "starting address"=u16 0, "Modbus master in"=w435) -> ("error out"=w432:errorcluster, "register values"=w389:u16[], "Modbus master out"=w433:refnum<class "Modbus Master.lvclass">)  [unwired: 5 in]
                    n601 = Index Array(array=w389, index #1=51 ("index"), index #2=52 ("index"), index #3=53 ("index"), index #4=54 ("index"), index #5=55 ("index"), index #6=56 ("index"), index #7=u16 44 ("address")) -> (element #1=w427:u16, element #2=w428:u16, element #3=w429:u16, element #4=w431:u16, element #5=w430:u16, element #6=w407:u16, element #7=w406:u16)
                    n602 = Index Array(array=w389, index #1=u16 22 ("address"), index #2=u16 57 ("address"), index #3=u16 21 ("address"), index #4=u16 58 ("address"), index #5=61 ("index")) -> (element #1=w453:u16, element #2=w450:u16, element #3=w447:u16, element #4=w444:u16, element #5=w440:u16)
                    n603 = Index Array(array=w389, index=u16 43 ("address")) -> (element=w387:u16)
                    n604 = Not Equal To 0?(x=w447) -> (x != 0?=w448:bool)
                    n605 = Index Array(array=w389, index #1=u16 14 ("address"), index #2=u16 15 ("address")) -> (element #1=w403:u16, element #2=w402:u16)
                    n606 = Not Equal To 0?(x=w453) -> (x != 0?=w454:bool)
                    n607 = Divide(x=w440, y=10.0) -> (x/y=w442:dbl)
                    n608 = Divide(x=w444, y=100.0) -> (x/y=w445:dbl)
                    n609 = Divide(x=w427, y=100.0) -> (x/y=w409:dbl)
                    n610 = Divide(x=w428, y=100.0) -> (x/y=w410:dbl)
                    n611 = Divide(x=w429, y=100.0) -> (x/y=w411:dbl)
                    n612 = Divide(x=w431, y=100.0) -> (x/y=w412:dbl)
                    n613 = Divide(x=w430, y=10.0) -> (x/y=w413:dbl)
                    n614 = Divide(x=w407, y=10.0) -> (x/y=w414:dbl)
                    n615 = Not Equal To 0?(x=w450) -> (x != 0?=w451:bool)
                    n616 = local write "Regulation TYpe"(w448) -> ()
                    n617 = Build Array(w403, w402) -> (w391:u16[])
                    n618 = local write "Heating Mode:"(w454) -> ()
                    n619 = local write "Target Ue [V]:"(w442) -> ()
                    n620 = local write "Target Ic [A]:"(w445) -> ()
                    n621 = local write "PID Output:"(w451) -> ()
                    n622 = local write "Ic limit [A]:"(w411) -> ()
                    n623 = local write "Ic limit:1"(w409) -> ()
                    n624 = local write "Uc limit:1"(w410) -> ()
                    n625 = local write "Uc limit [V]:"(w412) -> ()
                    n626 = local write "Ie limit [mA]:"(w413) -> ()
                    n627 = local write "Ue limit [V]:"(w414) -> ()
                    n628 = local write "Ramp unit:"(w406) -> ()
                    n629 = To Double Precision Float(number=w387) -> (double precision float=w386:dbl)
                    n630 = local read "Temp. unit:"() -> (w400:u16)
                    n631 = Type Cast(type=0, x=w391) -> (*(type *) &x=w399:i32)
                    n632 = To Double Precision Float(number=w399) -> (double precision float=w398:dbl)
                    n633 = Divide(x=w398, y=100.0) -> (x/y=w397:dbl)
                    n634 = Equal To 0?(x=w400) -> (x = 0?=w395:bool)
                    n635 = Divide(x=w386, y=10.0) -> (x/y=w385:dbl)
                    n636 = Subtract(x=w397, y=273.15) -> (x-y=w396:dbl)
                    n637 = local write "Target Ramp:"(w385) -> ()
                    n638 = Select(t=w396, s=w395, f=w397) -> (s? t:f=w401:dbl)
                    n639 = local write "Target Temp:"(w401) -> ()
                  }
                  frame Error {
                  }
                }
              }
              event "Ramp unit:": Value Change {
                n640 = event-data() -> ("NewVal"=w457:u16)  [unwired: 1 in, 5 out]
                n641 = call-dynamic "Write Single Holding Register.vi"("error in (no error)"=w458, "holding register value"=w457, "address"=u16 44, "Modbus master in"=w459) -> ("error out"=w460:errorcluster, "Modbus master out"=w461:refnum<class "Modbus Master.lvclass">)  [unwired: 6 in]
              }
              event "Ic limit:1": Value Change {
                n642 = event-data() -> ("NewVal"=w464:dbl)  [unwired: 1 in, 5 out]
                n643 = Multiply(x=w464, y=100.0) -> (x*y=w466:dbl)
                n644 = To Unsigned Word Integer(number=w466) -> (unsigned 16bit integer=w463:u16)
                n645 = call-dynamic "Write Single Holding Register.vi"("error in (no error)"=w467, "holding register value"=w463, "address"=u16 51, "Modbus master in"=w468) -> ("error out"=w469:errorcluster, "Modbus master out"=w470:refnum<class "Modbus Master.lvclass">)  [unwired: 6 in]
              }
              event "Uc limit:1": Value Change {
                n646 = event-data() -> ("NewVal"=w473:dbl)  [unwired: 1 in, 5 out]
                n647 = Multiply(x=w473, y=100.0) -> (x*y=w475:dbl)
                n648 = To Unsigned Word Integer(number=w475) -> (unsigned 16bit integer=w472:u16)
                n649 = call-dynamic "Write Single Holding Register.vi"("error in (no error)"=w476, "holding register value"=w472, "address"=u16 52, "Modbus master in"=w477) -> ("error out"=w478:errorcluster, "Modbus master out"=w479:refnum<class "Modbus Master.lvclass">)  [unwired: 6 in]
              }
              event "Ic limit [A]:": Value Change {
                n650 = event-data() -> ("NewVal"=w482:dbl)  [unwired: 1 in, 5 out]
                n651 = Multiply(x=w482, y=100.0) -> (x*y=w484:dbl)
                n652 = To Unsigned Word Integer(number=w484) -> (unsigned 16bit integer=w481:u16)
                n653 = call-dynamic "Write Single Holding Register.vi"("error in (no error)"=w485, "holding register value"=w481, "address"=u16 53, "Modbus master in"=w486) -> ("error out"=w487:errorcluster, "Modbus master out"=w488:refnum<class "Modbus Master.lvclass">)  [unwired: 6 in]
              }
              event "Uc limit [V]:": Value Change {
                n654 = event-data() -> ("NewVal"=w491:dbl)  [unwired: 1 in, 5 out]
                n655 = Multiply(x=w491, y=100.0) -> (x*y=w493:dbl)
                n656 = To Unsigned Word Integer(number=w493) -> (unsigned 16bit integer=w490:u16)
                n657 = call-dynamic "Write Single Holding Register.vi"("error in (no error)"=w494, "holding register value"=w490, "address"=u16 54, "Modbus master in"=w495) -> ("error out"=w496:errorcluster, "Modbus master out"=w497:refnum<class "Modbus Master.lvclass">)  [unwired: 6 in]
              }
              event "Ie limit [mA]:": Value Change {
                n658 = event-data() -> ("NewVal"=w500:dbl)  [unwired: 1 in, 5 out]
                n659 = Multiply(x=w500, y=10.0) -> (x*y=w502:dbl)
                n660 = To Unsigned Word Integer(number=w502) -> (unsigned 16bit integer=w499:u16)
                n661 = call-dynamic "Write Single Holding Register.vi"("error in (no error)"=w503, "holding register value"=w499, "address"=u16 55, "Modbus master in"=w504) -> ("error out"=w505:errorcluster, "Modbus master out"=w506:refnum<class "Modbus Master.lvclass">)  [unwired: 6 in]
              }
              event "Ue limit [V]:": Value Change {
                n662 = event-data() -> ("NewVal"=w509:dbl)  [unwired: 1 in, 5 out]
                n663 = Multiply(x=w509, y=10.0) -> (x*y=w511:dbl)
                n664 = To Unsigned Word Integer(number=w511) -> (unsigned 16bit integer=w508:u16)
                n665 = call-dynamic "Write Single Holding Register.vi"("error in (no error)"=w512, "holding register value"=w508, "address"=u16 56, "Modbus master in"=w513) -> ("error out"=w514:errorcluster, "Modbus master out"=w515:refnum<class "Modbus Master.lvclass">)  [unwired: 6 in]
              }
              event "Target Ue [V]:": Value Change {
                n666 = event-data() -> ("NewVal"=w518:dbl)  [unwired: 1 in, 5 out]
                n667 = Multiply(x=w518, y=10.0) -> (x*y=w520:dbl)
                n668 = To Unsigned Word Integer(number=w520) -> (unsigned 16bit integer=w517:u16)
                n669 = call-dynamic "Write Single Holding Register.vi"("error in (no error)"=w521, "holding register value"=w517, "address"=u16 61, "Modbus master in"=w522) -> ("error out"=w523:errorcluster, "Modbus master out"=w524:refnum<class "Modbus Master.lvclass">)  [unwired: 6 in]
              }
              event "Target Ic [A]:": Value Change {
                n670 = event-data() -> ("NewVal"=w527:dbl)  [unwired: 1 in, 5 out]
                n671 = Multiply(x=w527, y=100.0) -> (x*y=w529:dbl)
                n672 = To Unsigned Word Integer(number=w529) -> (unsigned 16bit integer=w526:u16)
                n673 = call-dynamic "Write Single Holding Register.vi"("error in (no error)"=w530, "holding register value"=w526, "address"=u16 58, "Modbus master in"=w531) -> ("error out"=w532:errorcluster, "Modbus master out"=w533:refnum<class "Modbus Master.lvclass">)  [unwired: 6 in]
              }
              event "Heating Mode:": Value Change {
                n674 = event-data() -> ("NewVal"=w536:bool)  [unwired: 1 in, 5 out]
                n675 = Boolean To (0,1)(Boolean=w536) -> (0, 1=w535:i16)
                n676 = To Unsigned Word Integer(number=w535) -> (unsigned 16bit integer=w537:u16)
                n677 = call-dynamic "Write Single Holding Register.vi"("error in (no error)"=w538, "holding register value"=w537, "address"=u16 22, "Modbus master in"=w539) -> ("error out"=w540:errorcluster, "Modbus master out"=w541:refnum<class "Modbus Master.lvclass">)  [unwired: 6 in]
              }
              event "Regulation TYpe": Value Change {
                n678 = event-data() -> ("NewVal"=w544:bool)  [unwired: 1 in, 5 out]
                n679 = Boolean To (0,1)(Boolean=w544) -> (0, 1=w543:i16)
                n680 = To Unsigned Word Integer(number=w543) -> (unsigned 16bit integer=w545:u16)
                n681 = call-dynamic "Write Single Holding Register.vi"("error in (no error)"=w546, "holding register value"=w545, "address"=u16 21, "Modbus master in"=w547) -> ("error out"=w548:errorcluster, "Modbus master out"=w549:refnum<class "Modbus Master.lvclass">)  [unwired: 6 in]
              }
              event "PID Output:": Value Change {
                n682 = event-data() -> ("NewVal"=w552:bool)  [unwired: 1 in, 5 out]
                n683 = Boolean To (0,1)(Boolean=w552) -> (0, 1=w551:i16)
                n684 = To Unsigned Word Integer(number=w551) -> (unsigned 16bit integer=w553:u16)
                n685 = call-dynamic "Write Single Holding Register.vi"("error in (no error)"=w554, "holding register value"=w553, "address"=u16 57, "Modbus master in"=w555) -> ("error out"=w556:errorcluster, "Modbus master out"=w557:refnum<class "Modbus Master.lvclass">)  [unwired: 6 in]
              }
              event "Target Temp:": Value Change {
                n686 = event-data() -> ("NewVal"=w575:dbl)  [unwired: 1 in, 5 out]
                n687 = local read "Temp. unit:"() -> (w559:u16)
                n688 = Add(x=w575, y=273.15) -> (x+y=w561:dbl)
                n689 = Equal To 0?(x=w559) -> (x = 0?=w562:bool)
                n690 = Select(t=w561, s=w562, f=w575) -> (s? t:f=w560:dbl)
                n691 = Multiply(x=w560, y=100.0) -> (x*y=w569:dbl)
                n692 = To Long Integer(number=w569) -> (32bit integer=w568:i32)
                n693 = Split Number(x=w568) -> (hi(x)=w567:u16, lo(x)=w566:u16)
                n694 = Build Array(w567, w566) -> (w564:u16[])
                n695 = call-dynamic "Write Multiple Holding Registers.vi"("error in (no error)"=w573, "holding register values"=w564, "starting address"=u16 14 ("address"), "Modbus master in"=w574) -> ("error out"=w571:errorcluster, "Modbus master out"=w572:refnum<class "Modbus Master.lvclass">)  [unwired: 6 in]
              }
              event "Target Ramp:": Value Change {
                n696 = event-data() -> ("NewVal"=w585:dbl)  [unwired: 1 in, 5 out]
                n697 = Multiply(x=w585, y=10.0) -> (x*y=w578:dbl)
                n698 = To Word Integer(number=w578) -> (16bit integer=w577:i16)
                n699 = Build Array(w577) -> (w576:i16[])
                n700 = call-dynamic "Write Multiple Holding Registers.vi"("error in (no error)"=w581, "holding register values"=w576, "starting address"=u16 43 ("address"), "Modbus master in"=w582) -> ("error out"=w583:errorcluster, "Modbus master out"=w584:refnum<class "Modbus Master.lvclass">)  [unwired: 6 in]
              }
            }
            n701 = local read "Remote:"() -> (w329:bool)
            n702 = case shown="True" w329 {
              tunnel: w334 -> [w355 w362]
              tunnel: [w355 w361] -> w333
              tunnel: "Lock Button" -> [_ w359]
              tunnel: w332 -> [w354 w357]
              tunnel: [w354 w356] -> w331
              frame False {
              }
              frame True {
                n703 = Boolean To (0,1)(Boolean=w359) -> (0, 1=w358:i16)
                n704 = call-dynamic "Write Single Holding Register.vi"("error in (no error)"=w357, "holding register value"=w358, "address"=1000 ("index"), "Modbus master in"=w362) -> ("error out"=w356:errorcluster, "Modbus master out"=w361:refnum<class "Modbus Master.lvclass">)  [unwired: 6 in]
              }
            }
          }
        }
        n705 = case shown="True" "Auto PID control:" {
          tunnel: "PID manual setting" -> [_ w675]
          tunnel: "PID auto tab" -> [w664 _]
          tunnel: [w655 w670] -> w228
          tunnel: [w654 w669] -> w227
          tunnel: [w653 w668] -> w226
          tunnel: w220 -> [w657 _]
          tunnel: [w651 0] -> w221
          frame False {
            n706 = Decimal String To Number(string=w664, default (0L)=0.0) -> (number=w659:dbl[][])  [unwired: 1 in, 1 out]
            n707 = Delete From Array(array=w659, index (col)=0 ("disabled index (col)")) -> (deleted portion=w656:dbl[], array with subset deleted=w658:dbl[][])  [unwired: 2 in]
            n708 = Threshold 1D Array(2:w657, 3:w656) -> (0:w652:dbl)  [unwired: 1 in]
            n709 = To Long Integer(number=w652) -> (32bit integer=w651:i32)
            n710 = Index Array(array=w658, index (row)=w651, index (col)=1 ("disabled index (col)")) -> (element=w654:dbl)
            n711 = Index Array(array=w658, index (row)=w651, index (col)=2 ("disabled index (col)")) -> (element=w653:dbl)
            n712 = Index Array(array=w658, index (row)=w651, index (col)=0 ("disabled index (col)")) -> (element=w655:dbl)
          }
          frame True {
            w671 = 0 ("disabled index (col)")
            n713 = Decimal String To Number(string=w675, default (0L)=0.0) -> (number=w667:dbl[][])  [unwired: 1 in, 1 out]
            n714 = Index Array(array=w667, index (row)=w671, index (col)=1 ("disabled index (col)")) -> (element=w669:dbl)
            n715 = Index Array(array=w667, index (row)=w671, index (col)=2 ("disabled index (col)")) -> (element=w668:dbl)
            n716 = Index Array(array=w667, index (row)=w671, index (col)=w671) -> (element=w670:dbl)
          }
        }
        "New P:" <- w228
        "New I:" <- w227
        "New D:" <- w226
        n717 = Bundle By Name(cluster=T13 {"Row"=0, "Column"=0} ("Selection Start"), "Row"=w221) -> (w222:T13)
        n718 = property on="PID auto tab" class="Tbl (strict)"("Selection Color"=u32 16860, "Selection Size"=T13 {"Row"=1, "Column"=4}, "Selection Start"=w222) -> ()  [unwired: 2 in, 2 out]
        n719 = Rotate 1D Array(1:w201, 2:1 ("n")) -> (0:w199:dbl[])
        n720 = Replace Array Subset(array=w199, new element=w187) -> (w198:dbl[])  [unwired: 1 in]
        n721 = Index Array(array=w198, index #1=0 ("n"), index #2=19 ("n")) -> (element #1=w194:dbl, element #2=w195:dbl)
        n722 = local read "Text Ring 3"() -> (w190:u16)
        "Text Ring 5" <- w190
        n723 = Subtract(x=w194, y=w195) -> (x-y=w193:dbl)
        n724 = Divide(x=w193, y=10.0) -> (x/y=w191:dbl)
        n725 = case shown="0, Default" w190 {
          tunnel: w191 -> [w233 w236 w240]
          tunnel: [w233 w234 w237] -> w189
          frame 0, Default {
            # "C/s"
          }
          frame 1 {
            # "C/m"
            n726 = Multiply(x=w236, y=60.0) -> (x*y=w234:dbl)
          }
          frame 2 {
            w238 = 60.0 ("y")
            # "C/h"
            n727 = Multiply(x=w240, y=w238) -> (x*y=w239:dbl)
            n728 = Multiply(x=w239, y=w238) -> (x*y=w237:dbl)
          }
        }
        "Act. Ramp:" <- w189
        n729 = local read "Boolean"() -> (w232:T2)
      }
      n730 = while {
        stop <- w169 stop-if-true
        # "XY Graph loop"
        n731 = case shown="True" "Start 3" {
          frame False {
          }
          frame True {
            n732 = property on="main Graph" class="WFChart (strict)"() -> ("History Data"=w172:T16)  [unwired: 2 in, 2 out]
            n733 = for {
              tunnel: w172 -> [w183] mode=indexing
              tunnel: [w182] -> w174 mode=indexing
              n734 = Cluster To Array(cluster=w183) -> (array=w182:dbl[])
            }
            n735 = Transpose 2D Array(2D array=w174) -> (transposed array=w170:dbl[][])
            n736 = Delete From Array(array=w170, index (row)=0) -> (deleted portion=w175:dbl[], array with subset deleted=w177:dbl[][])  [unwired: 2 in]
            n737 = Delete From Array(array=w177, index (row)=0) -> (array with subset deleted=w173:dbl[][])  [unwired: 2 in, 1 out]
            n738 = for {
              tunnel: w173 -> [w180] mode=indexing
              tunnel: w175 -> [w181]
              tunnel: [w179] -> w171 mode=indexing
              n739 = Bundle(w181, w180) -> (w179:cluster{dbl[], dbl[]})  [unwired: 1 in]
            }
            "XY Graph 2" <- w171
          }
        }
        n740 = Wait Until Next ms Multiple(millisecond multiple=u32 1000) -> ()  [unwired: 1 out]
        n741 = local read "Boolean"() -> (w169:T2)
      }
      n742 = local read "Connected:"() -> (w159:bool)
      n743 = case shown="True" w159 {
        tunnel: w165 -> [_ w185]
        tunnel: w164 -> [_ w184]
        frame False {
        }
        frame True {
          n744 = call "SRSRGAo Close.vi"("error in (no error)"=w184, "SRSRGA Refnum"=w185) -> ("error out"=w186:errorcluster)  [unwired: 9 in]
          n745 = call "SRSRGA Error Handler.vi"("error in (no error)"=w186) -> ()  [unwired: 9 in, 2 out]
        }
      }
      n746 = Compound Arithmetic op=AND(w152, w150, w151) -> (w166:bool)
      n747 = call-dynamic "Write Single Holding Register.vi"("error in (no error)"=w155, "holding register value"=u16 1, "address"=u16 71, "Modbus master in"=w156) -> ("error out"=w153:errorcluster, "Modbus master out"=w154:refnum<class "Modbus Master.lvclass">)  [unwired: 6 in]
      n748 = local write "stopped_loops"(w166) -> ()
      n749 = call-dynamic "Close.vi"("error in (no error)"=w153, "Modbus master in"=w154) -> ("error out"=w141:errorcluster)  [unwired: 9 in]
      n750 = call <vilib>:"Clear Errors.vi"("error in (no error)"=w141) -> ()  [unwired: 5 in, 2 out]
    }
    frame #2 {
      w1281 = "HEAT3 Sampling time"  # Key 1
      w1286 = "Recepice"  # Key 4
      w1296 = "HEAT3 PID manual tab"  # Key 3
      w1302 = "HEAT3 PID tab 1"  # Key 2
      w1285 = "Section 2"
      w1304 = "HEAT3 Path"  # Key 1
      w1278 = "Section 1"
      n751 = local read "PID manual setting"() -> (w1294:string[][])
      n752 = local read "Sampling time:"() -> (w1279:dbl)
      n753 = local read "PID auto tab"() -> (w1299:string[][])
      n754 = local read "Address:"() -> (w1303:string)
      n755 = property on="XY Graph" class="XYGraph (strict)"() -> ("CrsrList"=w1292:T22)  [unwired: 2 in, 2 out]
      n756 = call <vilib>:"Application Directory.vi"() -> ("Application Directory"=w1283:path)
      n757 = Build Path(base path=w1283, name or relative path="TDS Configuration File.ini") -> (appended path=w1282:path)
      n758 = Number To Fractional String(number=w1279) -> (F-format string=w1280:string)  [unwired: 3 in]
      n759 = Array To Spreadsheet String(array=w1299, 3:"%s" ("format string")) -> (spreadsheet string=w1301:string)  [unwired: 1 in]
      n760 = Array To Spreadsheet String(array=w1294, 3:"%s" ("format string")) -> (spreadsheet string=w1293:string)  [unwired: 1 in]
      n761 = Flatten To String(anything=w1292) -> (data string=w1287:string)  [unwired: 3 in, 2 out]
      n762 = Delete(path (use dialog)=w1282) -> (deleted path=w1307:path)  [unwired: 4 in, 2 out]
      n763 = call <vilib>:"Open Config Data.vi"("configuration file path"=w1307) -> ("error out"=w1305:errorcluster, "refnum"=w1306:T21)  [unwired: 2 in, 7 out]
      n764 = call-poly <vilib>:"Write Key.vi"("section"=w1278, "error in (no error)"=w1305, "value"=w1303, "key"=w1304, "refnum"=w1306) -> ("error out"=w1276:errorcluster, "refnum out"=w1277:T21)  [unwired: 1 in, 4 out]
      n765 = call-poly <vilib>:"Write Key.vi"("section"=w1278, "error in (no error)"=w1276, "value"=w1280, "key"=w1281, "refnum"=w1277) -> ("error out"=w1274:errorcluster, "refnum out"=w1275:T21)  [unwired: 1 in, 4 out]
      n766 = call-poly <vilib>:"Write Key.vi"("section"=w1285, "error in (no error)"=w1274, "value"=w1301, "key"=w1302, "refnum"=w1275) -> ("error out"=w1297:errorcluster, "refnum out"=w1298:T21)  [unwired: 1 in, 4 out]
      n767 = call-poly <vilib>:"Write Key.vi"("section"=w1285, "error in (no error)"=w1297, "value"=w1293, "key"=w1296, "refnum"=w1298) -> ("error out"=w1289:errorcluster, "refnum out"=w1291:T21)  [unwired: 1 in, 4 out]
      n768 = call-poly <vilib>:"Write Key.vi"("section"=w1285, "error in (no error)"=w1289, "value"=w1287, "key"=w1286, "refnum"=w1291) -> ("error out"=w1288:errorcluster, "refnum out"=w1290:T21)  [unwired: 1 in, 4 out]
      n769 = call <vilib>:"Close Config Data.vi"("error in (no error)"=w1288, "refnum"=w1290) -> ("error out"=w1273:errorcluster)  [unwired: 1 in, 8 out]
      n770 = call <vilib>:"Clear Errors.vi"("error in (no error)"=w1273) -> ()  [unwired: 5 in, 2 out]
    }
  }
  "Connected:" <- w13
  "Comunication error:" <- w13
